vi "COD主界面（列队使用）.vi"() -> (8 "多列列表框":i32(listbox))   [LabVIEW 2016, in "斯坦道CODMn.lvlib"]
uses:
  <vilib>/Plasmionique/MB Master/MB_Master_Serial/MB_Master_Serial.lvclass
  C:/Program Files (x86)/National Instruments/LabVIEW 2016/vi.lib/Plasmionique/MB Master/MB_Master/MB_Master.lvclass
  <vilib>/Analysis/6fits.llb/Curve Fitting Criteria.ctl
  <vilib>/Utility/miscctls.llb/LVPointTypeDef.ctl
  <vilib>/Utility/config.llb/Write Key (Double).vi
  <vilib>/Utility/config.llb/Read Key (Boolean).vi
  <vilib>/Utility/config.llb/Read Key (I32).vi
  <vilib>/Utility/config.llb/Read Key (Double).vi
  <vilib>/Utility/config.llb/Write Key (Boolean).vi
  <vilib>/Utility/config.llb/Write Key (I32).vi
  <vilib>/Waveform/WDTFileIO.llb/Read Waveform from File.vi
  <vilib>/Plasmionique/MB Master/MB Master.lvlib
  <vilib>/ptbypt/NI_PtbyPt.lvlib
  PLC/PLC.lvlib
  <vilib>/Utility/config.llb/NI_LVConfig.lvlib
  <vilib>/Analysis/NI_AALPro.lvlib
panel:
  in  "启用5":bool
  in  "校准5":bool
  in  "泵滴定数5":dbl
  in  "浓度5":dbl
  in  "启用4":bool
  in  "校准4":bool
  in  "泵滴定数4":dbl
  in  "浓度4":dbl
  out "波形时间":timestamp
  in  "历史波形":bool
  out "时间-ORP值":u16[](array[numeric]) caption="数组"
  out "ORP滴定曲线1":u16[](graph)
  out "滴定数-ORP值":u16[](array[numeric]) caption="数组"
  in  "关闭 3":bool
  in  "滴定曲线":bool
  out "ORP滴定曲线2":u16[](graph)
  in  "跨度液浓度":dbl
  out "空白测试标记":bool
  out "跨度核查标记":bool
  out "启动选择 2":u16(ring) items=["水样测试", "标样核查", "零点核查", "跨度核查", "空白测试", "加标回收", "平行样", "校零", "校标"]
  in  "量程选择":enum16{"低量程", "高量程"}(ring)
  out "MB_Serial session":refnum<class "MB_Master_Serial.lvclass">
  in  "手动控制":bool
  in  "选用水样":enum16{"葡萄糖", "草酸钠"}(ring)
  in  "方程系数":cluster{"X^2":dbl, "X":dbl, "b":dbl} {"X^2" format="%#.4g"; "b" format="%#.4g"; "X" format="%#.4g"}
  out "多项式系数1":dbl[](array[numeric]) caption="多项式系数"
  out "XY图":cluster{"X Values":dbl[], "Y Values":dbl[]}[](graph)
  in  "模型":enum32{"线性", "多项式"}(ring)
  out "启动时间":timestamp format="%<%Y/%m/%d %H:%M:%S>T"
  in  "自动切换量程":bool=TRUE
  in  "24H周期设置":bool[](xcontrol)
  in  "关闭 2":bool
  in  "周期设置":bool
  out "文本.文本":string
  out "r^2":dbl format="%.8g"
  out "拟合公式":string
  out "b":dbl format="%#.4g"
  out "K":dbl format="%#.4f"
  out "当前校准":i32
  in  "启用3":bool
  in  "启用2":bool
  in  "启用1":bool
  in  "校准3":bool
  in  "校准2":bool
  in  "校准1":bool
  in  "泵滴定数3":dbl
  in  "泵滴定数2":dbl
  in  "泵滴定数1":dbl
  in  "浓度3":dbl
  in  "浓度2":dbl
  in  "浓度1":dbl
  in  "写入":bool
  out "测量模式数字":i32
  out "零点核查标记":bool
  out "排液故障":bool
  out "进水样超量程":bool
  out "标样核查标记":bool
  out "平行样测量":bool
  out "加标回收测量":bool
  out "质控样测量":bool
  out "待机":bool
  out "校标错误":bool
  out "校零错误":bool
  out "测量错误":bool
  out "草酸钠报警":bool
  out "高锰酸钾报警":bool
  out "加热故障":bool
  out "温控器故障":bool
  out "ORP故障":bool
  out "排液标记":bool
  out "故障标记":bool
  out "校标标记":bool
  out "校零标记":bool
  out "通讯状态":bool
  out "水样测量":bool
  out "读取KB值":bool
  in  "读取":bool
  in  "返回":bool
  in  "校准配置":bool
  in  "修正系数 2":dbl
  in  "浓度 2":dbl
  in  "温度":dbl
  in  "恒温时间":dbl
  in  "基本量程":enum16{"10mL", "20mL"}(ring)
  in  "水样":dbl
  in  "蒸馏水":dbl
  in  "标液":dbl
  in  "质控样":dbl
  in  "加标回收":dbl
  in  "草酸钠":dbl
  in  "高锰酸钾":dbl
  in  "硫酸":dbl
  in  "零点泵计量数 2":dbl
  in  "标度泵计量数 2":dbl
  out "标度滴定值":dbl
  out "零点滴定值":dbl
  in  "保存":bool
  in  "关闭":bool
  out "测量数据区":T1 {"单位" items=["ug/L", "mg/L", "ppm", "mg/m3", "cm", "ppb", "ug/m3", "%", "nmol/mol", "umol/mol", "MPN/L", "MPN/100ml", "ng/m3", "NTU", "无量纲", "ms/cm", "us/cm", "℃", "mV", "万个/L"]}
  out "仪器时间":timestamp format="%<%Y/%m/%d %H:%M:%S>T"
  out "秒":u16
  out "分":u16
  out "COD浓度（mg/L)":dbl format="%.2g"
  out "进样管":dbl
  out "高锰酸钾":dbl
  out "草酸钠":dbl
  out "硫酸":dbl
  out "ORP显示":dbl
  out "温度":dbl
  out "加热":bool
  out "搅拌":bool
  out "进硫酸":bool
  out "进加标回收样":bool
  out "进质控样":bool
  out "进标液":bool
  out "进蒸馏水":bool
  out "进水样":bool
  out "进草酸钠":bool
  out "进高锰酸钾":bool
  in  "定时启动":bool
  in  "启动":bool
  in  "故障清除":bool
  in  "参数配置":bool
  in  "停止":bool
  in  "单步启动":bool
  out "定时时间":dbl
  out "系统时间":timestamp
  in  "时间校准":bool
  in  "枚举":enum16{"读取数据", "写入数据", "读取写入DATABASE", "读取参数"}(ring)
  in  "data in":T2
  out "报警簇":T3
  out "读取参数":u16[](array[numeric])
  out "DATABASE":u16[](array[numeric])
  out "Registers":u16[](array[numeric])
  in  "Slave ID":u8=1
  in  "Serial Config":T4={"baud rate (bps)"=115200, "stop bits"=10, "parity"=0, "flow control"=0, "timeout"=1000, "retries"=1} {"stop bits" items=["1.0"=10, "1.5"=15, "2.0"=20]; "flow control" items=["None", "XON/XOFF", "RTS/CTS", "XON/XOFF & RTS/CTS", "DTR/DSR", "XON/XOFF & DTR/DSR"]; "parity" items=["None", "Odd", "Even", "Mark", "Space"]}
  out "table 输入":string
  out "columns":string[](array[string])
  out "data":T5
  in  "温度 2":dbl
  in  "浓度":dbl
  in  "修正系数":dbl
  in  "标样浓度 2":dbl
  out "模式（受控）":u16
  in  "VISA resource name":refnum<visa-resource-name>="COM4" caption="VISA资源名称"
  # "测量时间："
  # "水样~加标回收"
  # "mV"
  # "℃"
  # "注：遇到加热故障和排液故障时仪器不能正常启动，\n必须排查故障并点击报警清除按钮方可运行。"
  # "mg/L"
  # "校零校标结果"
  # "基本参数设置"
  # "泵计量参数设置"
  # "校零结果："
  # "校零滴定值："
  # "加热恒温温度（℃）："
  # "水样："
  # "高锰酸钾："
  # "校标结果："
  # "标度滴定值："
  # "零点泵计量值："
  # "恒温时间（分钟）："
  # "蒸馏水："
  # "草酸钠："
  # "标度泵计量值："
  # "标准液浓度（mg/L）："
  # "标液："
  # "标样浓度："
  # "硫酸："
  # "修正系数："
  # "质控样："
  # "跨度液浓度："
  # "基本量程（20mL可选）："
  # "加标回收样："
  # "是否启用"
  # "泵滴定数"
  # "浓度"
  # "辅\n助\n计\n算\n区"
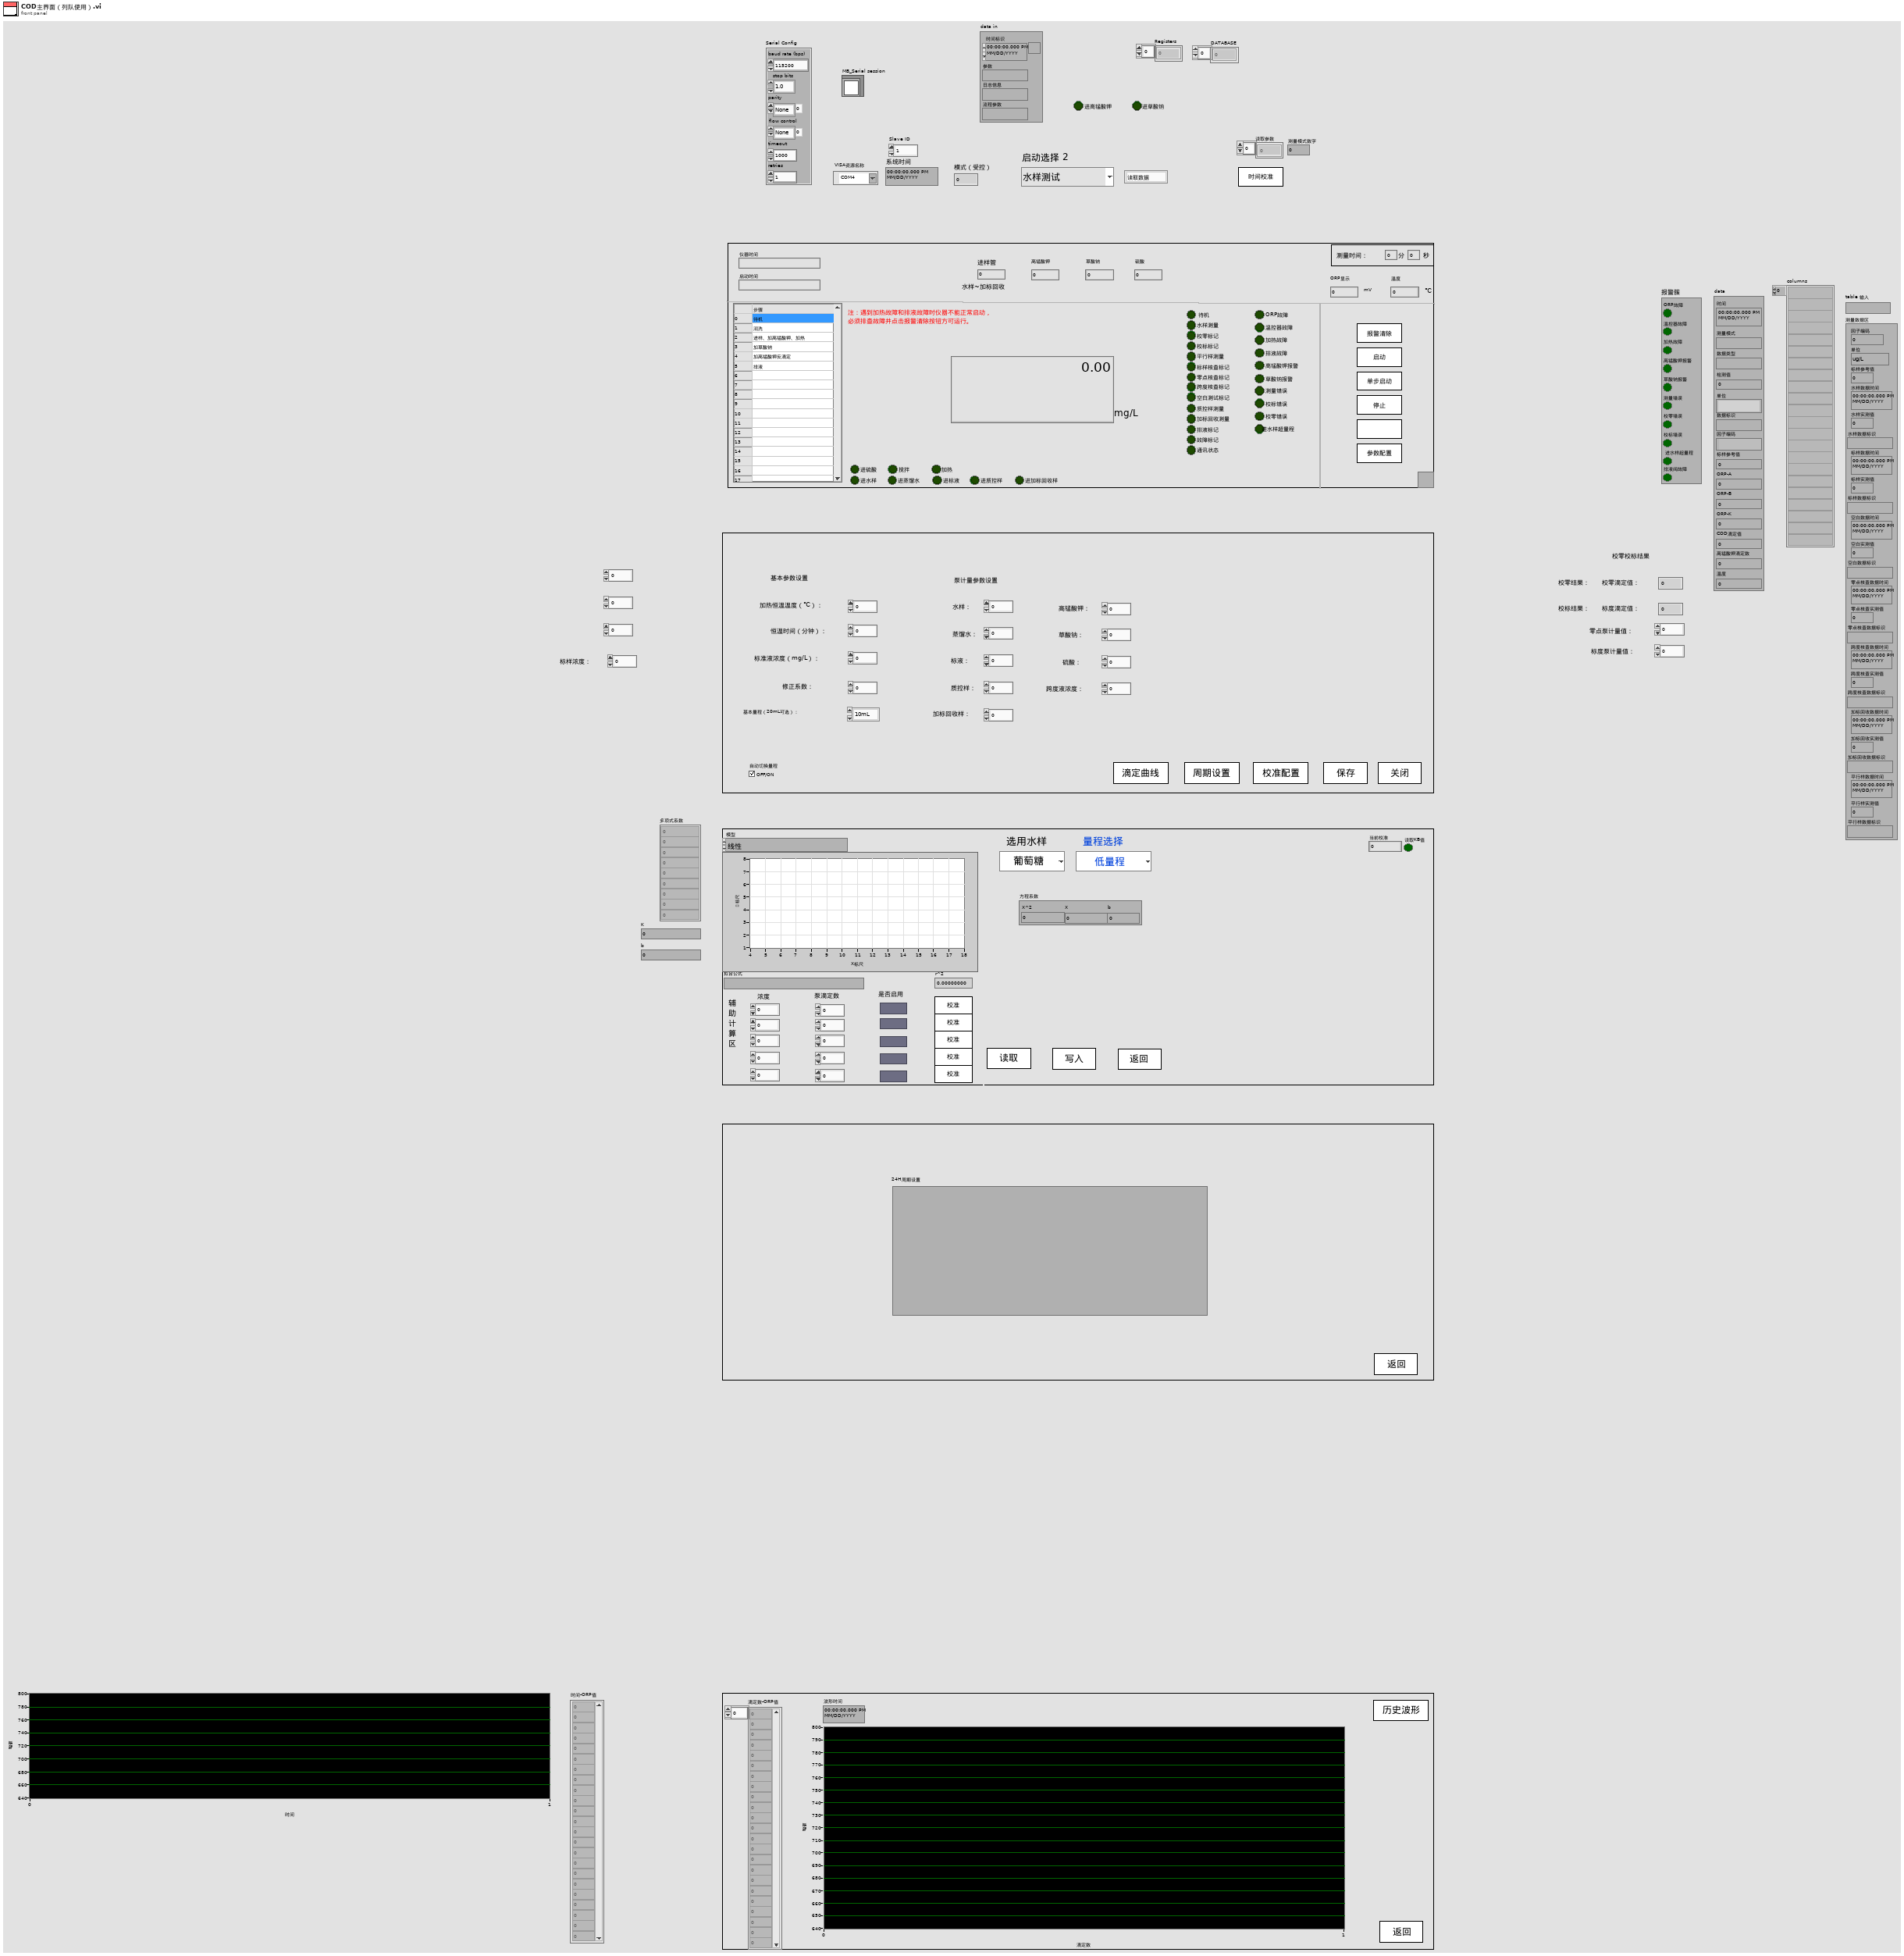
[diagram p1: front panel]
types:
  T1 = cluster{"因子编码":u32, "单位":u16, "标样参考值":sgl, "水样数据时间":timestamp, "水样实测值":sgl, "水样数据标识":string, "标样数据时间":timestamp, "标样实测值":sgl, "标样数据标识":string, "空白数据时间":timestamp, "空白实测值":sgl, "空白数据标识":string, "零点核查数据时间":timestamp, "零点核查实测值":sgl, "零点核查数据标识":string, "跨度核查数据时间":timestamp, "跨度核查实测值":sgl, "跨度核查数据标识":string, "加标回收数据时间":timestamp, "加标回收实测值":sgl, "加标回收数据标识":string, "平行样数据时间":timestamp, "平行样实测值":sgl, "平行样数据标识":string}
  T2 = cluster{"时间标识":timestamp, "参数":string, "日志信息":string, "流程参数":string}
  T3 = cluster{"ORP故障":bool, "温控器故障":bool, "加热故障":bool, "高锰酸钾报警":bool, "草酸钠报警":bool, "测量错误":bool, "校零错误":bool, "校标错误":bool, " 进水样超量程":bool, "排液阀故障":bool}
  T4 = cluster{"baud rate (bps)":u32, "stop bits":u16, "parity":u16, "flow control":u16, "timeout":u32, "retries":i32}
  T5 = cluster{"时间":timestamp, "测量模式":string, "数据类型":string, "检测值":sgl, "单位":string, "数据标识":string, "因子编码":string, "标样参考值":sgl, "ORP-A":sgl, "ORP-B":sgl, "ORP-K":sgl, "COD滴定值":sgl, "高锰酸钾滴定数":sgl, "温度":sgl}
  T6 = cluster{"starting address":u16, "number of holding registers":u16}
  T7 = cluster{"测量模式":enum16{"水样测量", "标样核查", "零点核查", "跨度核查", "空白测试", "加标回收", "平行样", "校零", "校标"}}
  T8 = typedef "LVDateTimeRec.ctl" = cluster{"秒数的小数部分":dbl, "秒":i32, "分":i32, "时":i32, "日":i32, "月":i32, "年":i32, "天数（周）":i32, "天数（年）":i32, "DST":i32}
  T9 = typedef "LVPointTypeDef.ctl" = cluster{"Horizontal":i16, "Vertical":i16}
  T10 = typedef "NI_LVConfig.lvlib/Config Data RefNum.ctl" = refnum<k1>
  T11 = cluster{"时间标识":timestamp, "设备":string, "日志信息":string}
  T12 = typedef "NI_AALPro.lvlib/Curve Fitting Criteria.ctl" = u16
  T13 = cluster{"时间标识":timestamp, "设备":string, "日志信息":string, "流程参数":string}
  T14 = cluster{"数组 2[0]":sgl, "数组 2[1]":sgl, "数组 2[2]":sgl, "数组 2[3]":sgl, "数组 2[4]":sgl, "数组 2[5]":sgl}
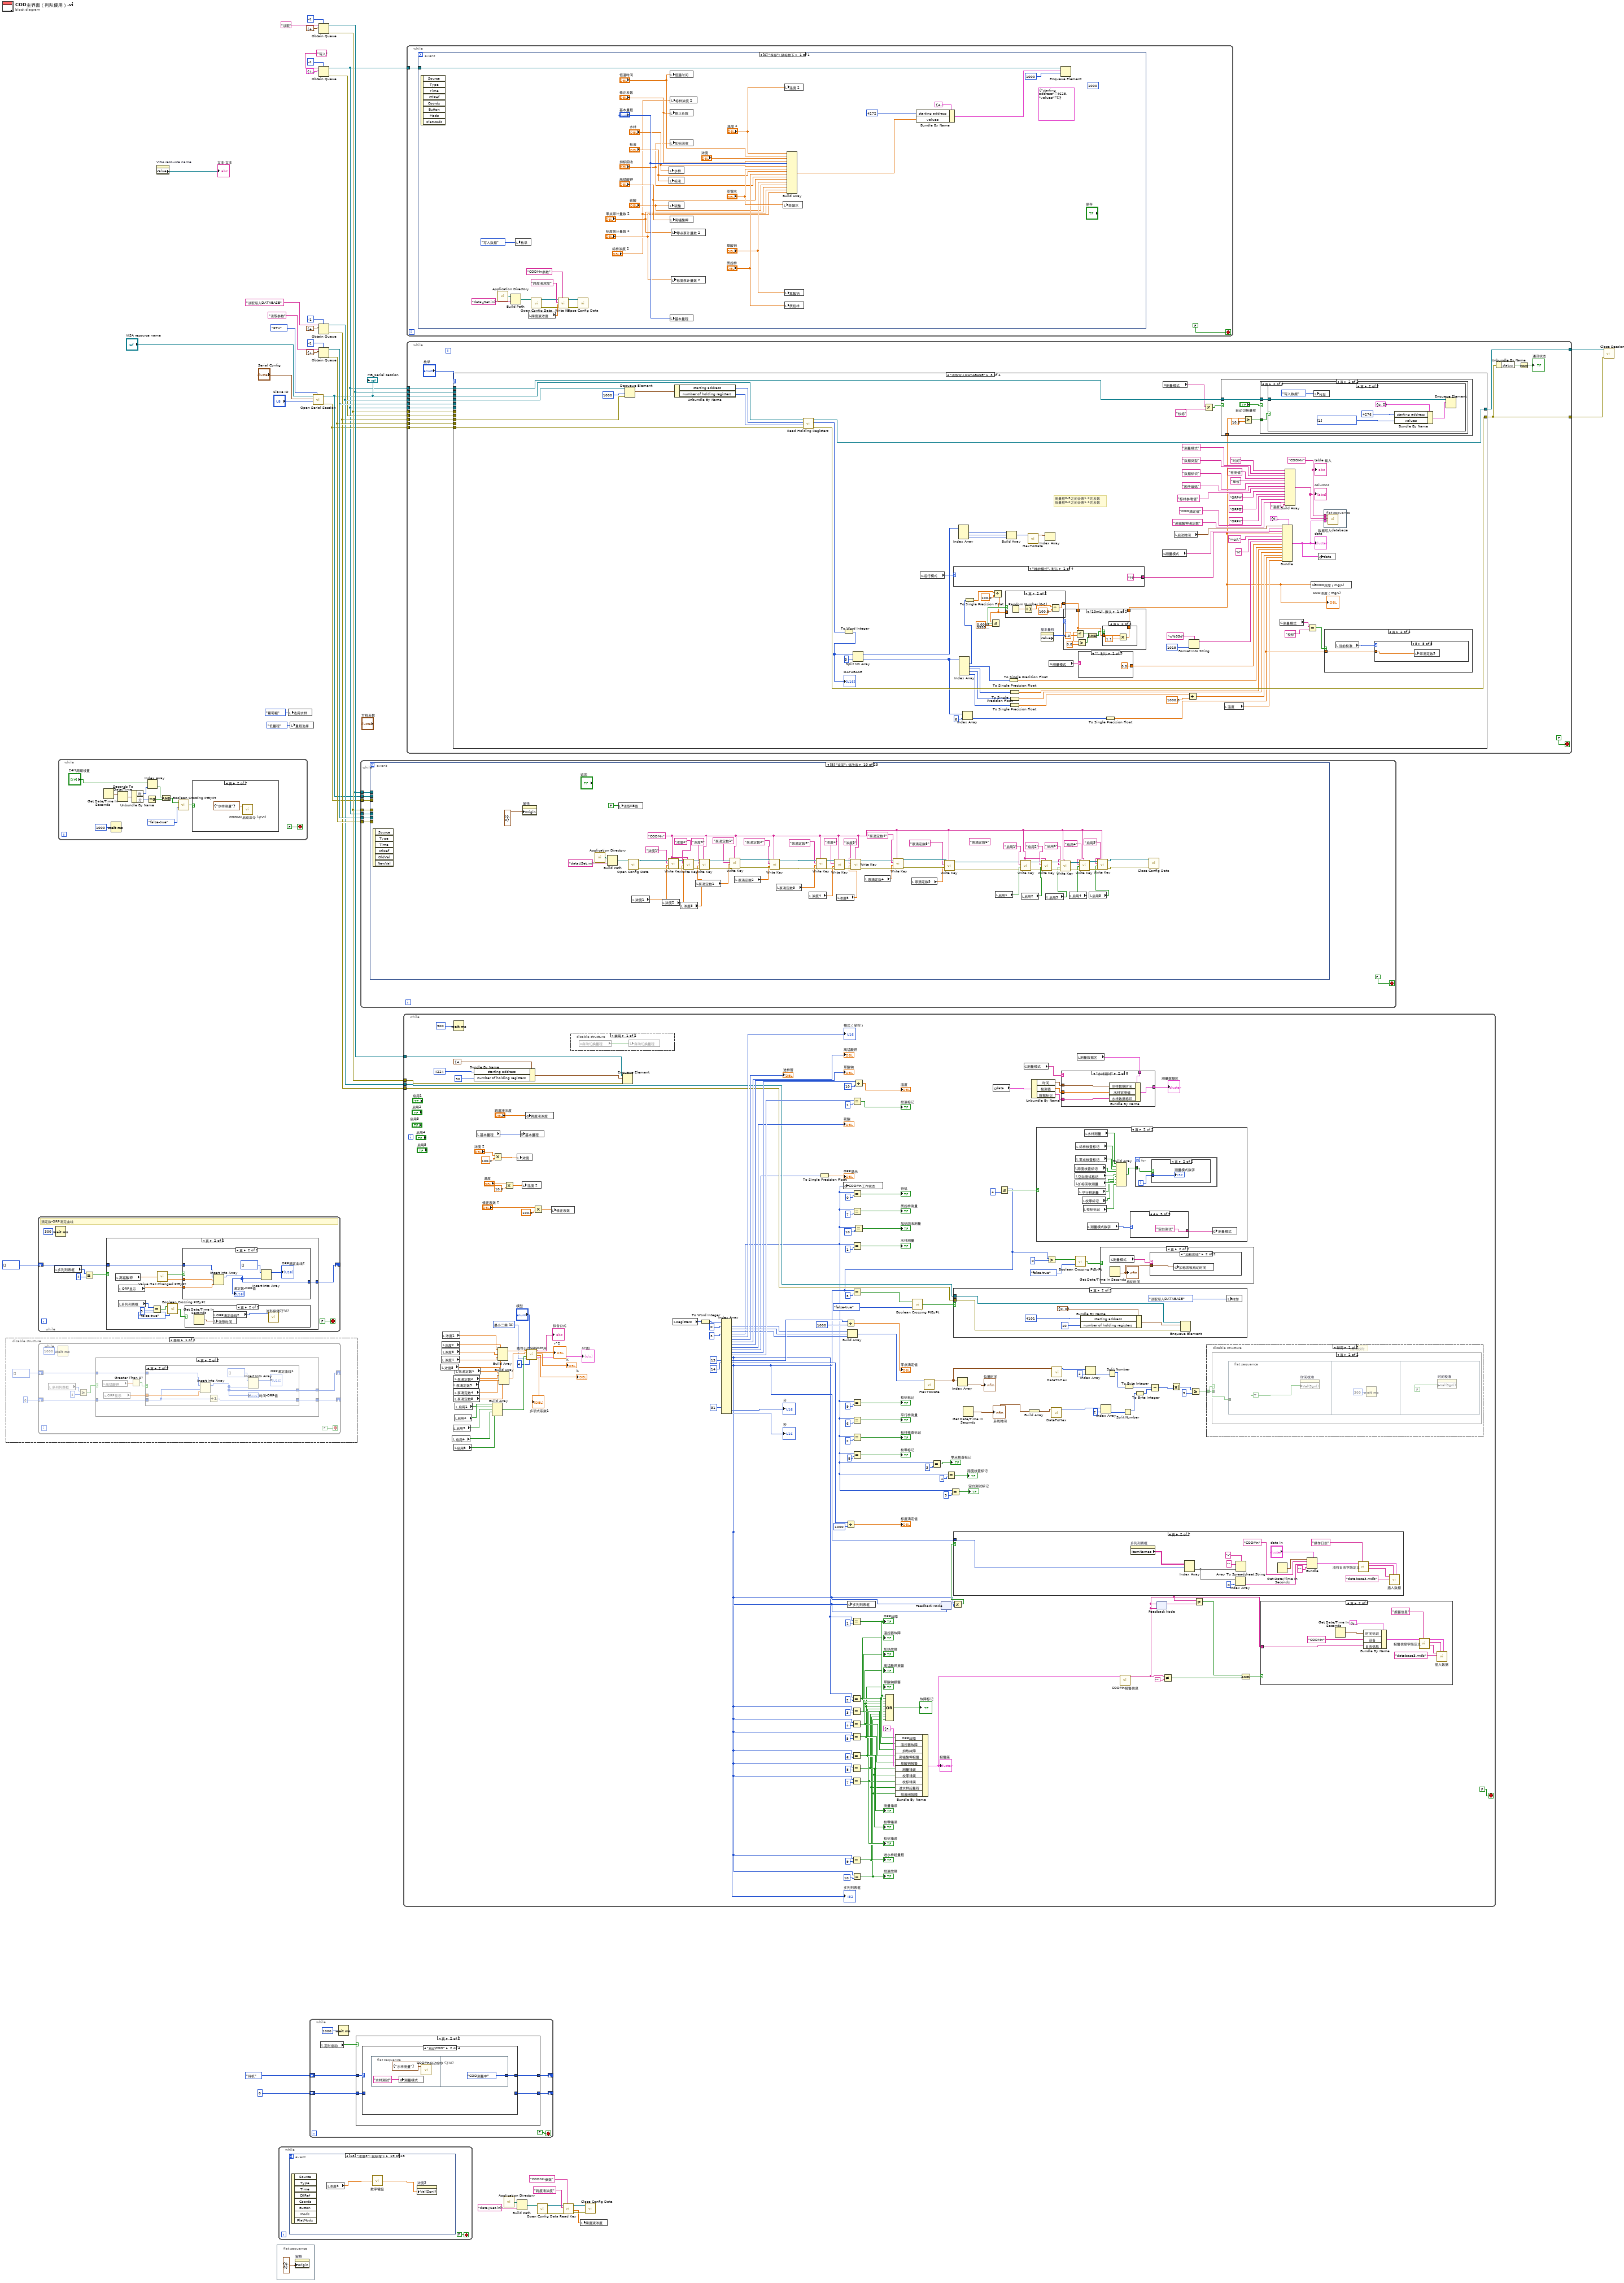
[diagram p0: block diagram]
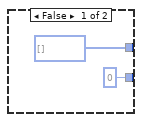
[diagram p2: hidden frame]
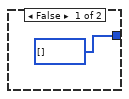
[diagram p5: hidden frame]
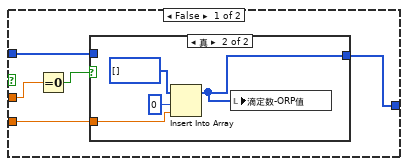
[diagram p7: hidden frame]
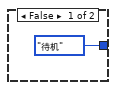
[diagram p10: hidden frame]
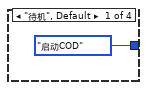
[diagram p11: hidden frame]
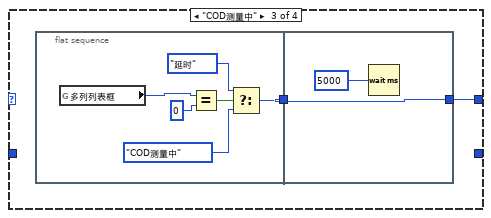
[diagram p12: hidden frame]
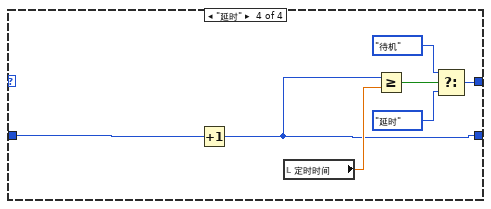
[diagram p13: hidden frame]
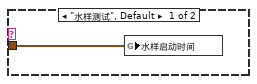
[diagram p18: hidden frame]
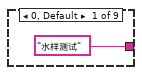
[diagram p20: hidden frame]
diagram:
  n1 = disable-structure shown="禁用" {
    frame Disabled {
      n2 = while {
        shift-right: [w49] -> _
        shift-left: u16[] [] ("ORP滴定曲线") -> [w51]
        shift-right: [w48] -> _
        shift-left: 0 -> [w50]
        stop <- FALSE stop-if-true
        n3 = local read "多列列表框"() -> (w53:i32)
        n4 = Wait (ms)(milliseconds to wait=u32 1000 ("等待时间（毫秒）")) -> ()  [unwired: 1 out]
        n5 = Greater Or Equal?(x=w53, y=4) -> (x >= y?=w52:bool)
        n6 = case shown="真" w52 {
          tunnel: w51 -> [_ w63]
          tunnel: w50 -> [_ w61]
          tunnel: [u16[] [] ("ORP滴定曲线") w59] -> w49
          tunnel: [0 w58] -> w48
          frame False {
          }
          frame True {
            n7 = local read "高锰酸钾"() -> (w62:dbl)
            n8 = local read "ORP显示"() -> (w60:dbl)
            n9 = Greater Than 0?(x=w62) -> (x > 0?=w64:bool)
            n10 = case shown="真" w64 {
              tunnel: w63 -> [w65 w72]
              tunnel: w61 -> [w66 w69]
              tunnel: w60 -> [_ w71]
              tunnel: [w65 w70] -> w59
              tunnel: [w66 w68] -> w58
              frame False {
              }
              frame True {
                n11 = Insert Into Array(array=w72, index=w69, new element=w71) -> (w70:u16[])
                "时间-ORP值" <- w70
                n12 = Increment(x=w69) -> (x+1=w68:i32)
                n13 = Insert Into Array(array=u16[] [] ("ORP滴定曲线"), new element=w70) -> (→"ORP滴定曲线1":u16[])  [unwired: 1 in]
              }
            }
          }
        }
      }
    }
    frame Enabled {
    }
  }
  n14 = while {
    shift-right: [w77] -> _
    shift-left: u16[] [] ("ORP滴定曲线") -> [w78]
    stop <- FALSE stop-if-true
    # "滴定数-ORP滴定曲线"
    n15 = local read "多列列表框"() -> (w76:i32)
    n16 = Wait (ms)(milliseconds to wait=u32 300 ("等待时间（毫秒）")) -> ()  [unwired: 1 out]
    n17 = Greater Or Equal?(x=w76, y=4) -> (x >= y?=w74:bool)
    n18 = case shown="真" w74 {
      tunnel: w78 -> [_ w92]
      tunnel: [u16[] [] ("ORP滴定曲线") w91] -> w77
      frame False {
      }
      frame True {
        n19 = local read "高锰酸钾"() -> (w88:dbl)
        n20 = local read "多列列表框"() -> (w86:i32)
        n21 = local read "ORP显示"() -> (w87:dbl)
        n22 = Equal?(x=w86, y=5) -> (x = y?=w84:bool)
        n23 = call <vilib>:"Value Has Changed PtByPt.vi"("input data point"=w88) -> ("has changed"=w90:bool, "output data point"=w89:dbl)  [unwired: 1 in]
        n24 = call <vilib>:"Boolean Crossing PtByPt.vi"("direction"=enum16{"either", "false-true", "true-false"}."false-true", "input"=w84) -> ("crossing"=w82:bool)  [unwired: 1 in]
        n25 = case shown="真" w90 {
          tunnel: w92 -> [w98 w108]
          tunnel: [w97 w107] -> w91
          tunnel: w89 -> [w99 w106]
          tunnel: w87 -> [w95 w105]
          frame False {
            n26 = Equal To 0?(x=w99) -> (x = 0?=w96:bool)
            n27 = case shown="真" w96 {
              tunnel: [w100 w103] -> w97
              tunnel: w98 -> [w100 _]
              tunnel: w95 -> [_ w102]
              frame False {
              }
              frame True {
                n28 = Insert Into Array(array=u16[] [] ("ORP滴定曲线"), index=0 ("索引"), new element=w102) -> (w103:u16[])
                n29 = local write "滴定数-ORP值"(w103) -> ()
              }
            }
          }
          frame True {
            n30 = Insert Into Array(array=w108, index=w106, new element=w105) -> (w107:u16[])
            "滴定数-ORP值" <- w107
            n31 = Insert Into Array(array=u16[] [] ("ORP滴定曲线"), new element=w107) -> (→"ORP滴定曲线2":u16[])  [unwired: 1 in]
          }
        }
        n32 = case shown="真" w82 {
          frame False {
          }
          frame True {
            n33 = Get Date/Time In Seconds() -> (seconds since 1Jan1904=w93:timestamp)
            n34 = local read "ORP滴定曲线2"() -> (w94:u16[])
            n35 = local write "波形时间"(w93) -> ()
            n36 = call "波形存储(子VI).vi"("ORP滴定曲线"=w94) -> ()  [unwired: 11 in]
          }
        }
      }
    }
  }
  n37 = while {
    stop <- FALSE stop-if-true
    n38 = Get Date/Time In Seconds() -> (seconds since 1Jan1904=w122:timestamp)
    n39 = Wait (ms)(milliseconds to wait=u32 1000 ("等待时间（毫秒）")) -> ()  [unwired: 1 out]
    n40 = Seconds To Date/Time(time stamp (now)=w122) -> (date time rec=w121:T8)  [unwired: 1 in]
    n41 = Unbundle By Name(w121) -> ("时"=w118:i32, "分"=w120:i32)
    n42 = Equal To 0?(x=w120) -> (x = 0?=w119:bool)
    n43 = Index Array(array="24H周期设置", index=w118) -> (element=w117:bool)
    n44 = And(x=w117, y=w119) -> (x .and. y?=w115:bool)
    n45 = call <vilib>:"Boolean Crossing PtByPt.vi"("direction"=enum16{"either", "false-true", "true-false"}."false-true", "input"=w115) -> ("crossing"=w114:bool)  [unwired: 1 in]
    n46 = case shown="真" w114 {
      frame False {
      }
      frame True {
        n47 = call "CODMn启动命令 (子VI).vi"("启动测量模式"=T7 {"测量模式"=enum."水样测量"}) -> ()  [unwired: 11 in]
      }
    }
  }
  n48 = property on="VISA resource name" class="VISAName"() -> ("Value"=→"文本.文本":refnum<visa-resource-name>)  [unwired: 2 in, 2 out]
  n49 = flat-sequence {
    frame #0 {
      n50 = property on="窗格" class="Pane"("Origin"=T9 {"Horizontal"=0, "Vertical"=0} ("原点")) -> ()  [unwired: 2 in, 2 out]
    }
  }
  n51 = while {
    stop <- FALSE stop-if-true
    n52 = event shown="[18] \"浓度3\": 鼠标按下" {
      selector: _ -> [_ _ _ _ _ _ _ _ _ _ _ _ _ _ _ _ _ _ _ _ _ _ _ _ _ _ _ _]
      dyn-events: _ -> [_ _ _ _ _ _ _ _ _ _ _ _ _ _ _ _ _ _ _ _ _ _ _ _ _ _ _ _]
      timeout: _ -> [_ _ _ _ _ _ _ _ _ _ _ _ _ _ _ _ _ _ _ _ _ _ _ _ _ _ _ _]
      event Timeout {
        n53 = event-data() -> ()  [unwired: 1 in, 3 out]
      }
      event "温度": Mouse Down {
        n54 = event-data() -> ()  [unwired: 1 in, 8 out]
        n55 = local read "温度"() -> (w127:dbl)
        n56 = call "数字键盘.vi"("OldNumber"=w127) -> ("NewNumber"=w126:sgl)
        n57 = local write "温度"(w126) -> ()
      }
      event "恒温时间": Mouse Down {
        n58 = event-data() -> ()  [unwired: 1 in, 8 out]
        n59 = local read "恒温时间"() -> (w128:dbl)
        n60 = call "数字键盘.vi"("OldNumber"=w128) -> ("NewNumber"=w129:sgl)
        n61 = local write "恒温时间"(w129) -> ()
      }
      event "浓度 2": Mouse Down {
        n62 = event-data() -> ()  [unwired: 1 in, 8 out]
        n63 = local read "浓度 2"() -> (w131:dbl)
        n64 = call "数字键盘.vi"("OldNumber"=w131) -> ("NewNumber"=w130:sgl)
        n65 = local write "浓度 2"(w130) -> ()
      }
      event "修正系数 2": Mouse Down {
        n66 = event-data() -> ()  [unwired: 1 in, 8 out]
        n67 = local read "修正系数 2"() -> (w132:dbl)
        n68 = call "数字键盘.vi"("OldNumber"=w132) -> ("NewNumber"=w133:sgl)
        n69 = local write "修正系数 2"(w133) -> ()
      }
      event "水样": Mouse Down {
        n70 = event-data() -> ()  [unwired: 1 in, 8 out]
        n71 = local read "水样"() -> (w134:dbl)
        n72 = call "数字键盘.vi"("OldNumber"=w134) -> ("NewNumber"=w135:sgl)
        n73 = local write "水样"(w135) -> ()
      }
      event "蒸馏水": Mouse Down {
        n74 = event-data() -> ()  [unwired: 1 in, 8 out]
        n75 = local read "蒸馏水"() -> (w136:dbl)
        n76 = call "数字键盘.vi"("OldNumber"=w136) -> ("NewNumber"=w137:sgl)
        n77 = local write "蒸馏水"(w137) -> ()
      }
      event "标液": Mouse Down {
        n78 = event-data() -> ()  [unwired: 1 in, 8 out]
        n79 = local read "标液"() -> (w138:dbl)
        n80 = call "数字键盘.vi"("OldNumber"=w138) -> ("NewNumber"=w139:sgl)
        n81 = local write "标液"(w139) -> ()
      }
      event "质控样": Mouse Down {
        n82 = event-data() -> ()  [unwired: 1 in, 8 out]
        n83 = local read "质控样"() -> (w140:dbl)
        n84 = call "数字键盘.vi"("OldNumber"=w140) -> ("NewNumber"=w141:sgl)
        n85 = local write "质控样"(w141) -> ()
      }
      event "加标回收": Mouse Down {
        n86 = event-data() -> ()  [unwired: 1 in, 8 out]
        n87 = local read "加标回收"() -> (w142:dbl)
        n88 = call "数字键盘.vi"("OldNumber"=w142) -> ("NewNumber"=w143:sgl)
        n89 = local write "加标回收"(w143) -> ()
      }
      event "草酸钠": Mouse Down {
        n90 = event-data() -> ()  [unwired: 1 in, 8 out]
        n91 = local read "草酸钠"() -> (w144:dbl)
        n92 = call "数字键盘.vi"("OldNumber"=w144) -> ("NewNumber"=w145:sgl)
        n93 = local write "草酸钠"(w145) -> ()
      }
      event "高锰酸钾": Mouse Down {
        n94 = event-data() -> ()  [unwired: 1 in, 8 out]
        n95 = local read "高锰酸钾"() -> (w146:dbl)
        n96 = call "数字键盘.vi"("OldNumber"=w146) -> ("NewNumber"=w147:sgl)
        n97 = local write "高锰酸钾"(w147) -> ()
      }
      event "硫酸": Mouse Down {
        n98 = event-data() -> ()  [unwired: 1 in, 8 out]
        n99 = local read "硫酸"() -> (w148:dbl)
        n100 = call "数字键盘.vi"("OldNumber"=w148) -> ("NewNumber"=w149:sgl)
        n101 = local write "硫酸"(w149) -> ()
      }
      event "零点泵计量数 2": Mouse Down {
        n102 = event-data() -> ()  [unwired: 1 in, 8 out]
        n103 = local read "零点泵计量数 2"() -> (w150:dbl)
        n104 = call "数字键盘.vi"("OldNumber"=w150) -> ("NewNumber"=w151:sgl)
        n105 = local write "零点泵计量数 2"(w151) -> ()
      }
      event "标度泵计量数 2": Mouse Down {
        n106 = event-data() -> ()  [unwired: 1 in, 8 out]
        n107 = local read "标度泵计量数 2"() -> (w152:dbl)
        n108 = call "数字键盘.vi"("OldNumber"=w152) -> ("NewNumber"=w153:sgl)
        n109 = local write "标度泵计量数 2"(w153) -> ()
      }
      event "标样浓度 2": Mouse Down {
        n110 = event-data() -> ()  [unwired: 1 in, 8 out]
        n111 = local read "标样浓度 2"() -> (w154:dbl)
        n112 = call "数字键盘.vi"("OldNumber"=w154) -> ("NewNumber"=w155:sgl)
        n113 = local write "标样浓度 2"(w155) -> ()
      }
      event "浓度1": Mouse Down {
        n114 = event-data() -> ()  [unwired: 1 in, 8 out]
        n115 = local read "浓度1"() -> (w157:dbl)
        n116 = call "数字键盘.vi"("OldNumber"=w157) -> ("NewNumber"=w156:sgl)
        n117 = property on="浓度1" class="DigNum (严格)"("Val(Sgnl)"=w156) -> ()  [unwired: 2 in, 2 out]
      }
      event "浓度2": Mouse Down {
        n118 = event-data() -> ()  [unwired: 1 in, 8 out]
        n119 = local read "浓度2"() -> (w159:dbl)
        n120 = call "数字键盘.vi"("OldNumber"=w159) -> ("NewNumber"=w158:sgl)
        n121 = property on="浓度2" class="DigNum (严格)"("Val(Sgnl)"=w158) -> ()  [unwired: 2 in, 2 out]
      }
      event "浓度3": Mouse Down {
        n122 = event-data() -> ()  [unwired: 1 in, 8 out]
        n123 = local read "浓度3"() -> (w161:dbl)
        n124 = call "数字键盘.vi"("OldNumber"=w161) -> ("NewNumber"=w160:sgl)
        n125 = property on="浓度3" class="DigNum (严格)"("Val(Sgnl)"=w160) -> ()  [unwired: 2 in, 2 out]
      }
      event "浓度4": Mouse Down {
        n126 = event-data() -> ()  [unwired: 1 in, 8 out]
        n127 = local read "浓度4"() -> (w163:dbl)
        n128 = call "数字键盘.vi"("OldNumber"=w163) -> ("NewNumber"=w162:sgl)
        n129 = property on="浓度4" class="DigNum (严格)"("Val(Sgnl)"=w162) -> ()  [unwired: 2 in, 2 out]
      }
      event "浓度5": Mouse Down {
        n130 = event-data() -> ()  [unwired: 1 in, 8 out]
        n131 = local read "浓度5"() -> (w165:dbl)
        n132 = call "数字键盘.vi"("OldNumber"=w165) -> ("NewNumber"=w164:sgl)
        n133 = property on="浓度5" class="DigNum (严格)"("Val(Sgnl)"=w164) -> ()  [unwired: 2 in, 2 out]
      }
      event "跨度液浓度": Mouse Down {
        n134 = event-data() -> ()  [unwired: 1 in, 8 out]
        n135 = local read "跨度液浓度"() -> (w167:dbl)
        n136 = call "数字键盘.vi"("OldNumber"=w167) -> ("NewNumber"=w166:sgl)
        n137 = property on="跨度液浓度" class="DigNum (严格)"("Val(Sgnl)"=w166) -> ()  [unwired: 2 in, 2 out]
      }
      event "跨度液浓度": Value Change {
        n138 = event-data() -> ()  [unwired: 1 in, 6 out]
        n139 = call <vilib>:"Application Directory.vi"() -> ("Application Directory"=w171:path)
        n140 = Build Path(base path=w171, name or relative path="data\\Set.ini" ("名称或相对路径")) -> (appended path=w173:path)
        n141 = local read "跨度液浓度"() -> (w168:dbl)
        n142 = call <vilib>:"Open Config Data.vi"("configuration file path"=w173) -> ("error out"=w175:errorcluster, "refnum"=w174:T10)  [unwired: 8 in, 1 out]
        n143 = call-poly <vilib>:"Write Key.vi"("section"="CODMn参数" ("key"), "error in (no error)"=w175, "value"=w168, "key"="跨度液浓度", "refnum"=w174) -> ("error out"=w177:errorcluster, "refnum out"=w176:T10)  [unwired: 4 in, 1 out]
        n144 = call <vilib>:"Close Config Data.vi"("error in (no error)"=w177, "refnum"=w176) -> ()  [unwired: 8 in, 2 out]
      }
      event "泵滴定数1": Mouse Down {
        n145 = event-data() -> ()  [unwired: 1 in, 8 out]
        n146 = local read "泵滴定数1"() -> (w179:dbl)
        n147 = call "数字键盘.vi"("OldNumber"=w179) -> ("NewNumber"=w178:sgl)
        n148 = property on="泵滴定数1" class="DigNum (严格)"("Val(Sgnl)"=w178) -> ()  [unwired: 2 in, 2 out]
      }
      event "泵滴定数2": Mouse Down {
        n149 = event-data() -> ()  [unwired: 1 in, 8 out]
        n150 = local read "泵滴定数2"() -> (w181:dbl)
        n151 = call "数字键盘.vi"("OldNumber"=w181) -> ("NewNumber"=w180:sgl)
        n152 = property on="泵滴定数2" class="DigNum (严格)"("Val(Sgnl)"=w180) -> ()  [unwired: 2 in, 2 out]
      }
      event "泵滴定数3": Mouse Down {
        n153 = event-data() -> ()  [unwired: 1 in, 8 out]
        n154 = local read "泵滴定数3"() -> (w183:dbl)
        n155 = call "数字键盘.vi"("OldNumber"=w183) -> ("NewNumber"=w182:sgl)
        n156 = property on="泵滴定数3" class="DigNum (严格)"("Val(Sgnl)"=w182) -> ()  [unwired: 2 in, 2 out]
      }
      event "泵滴定数4": Mouse Down {
        n157 = event-data() -> ()  [unwired: 1 in, 8 out]
        n158 = local read "泵滴定数4"() -> (w185:dbl)
        n159 = call "数字键盘.vi"("OldNumber"=w185) -> ("NewNumber"=w184:sgl)
        n160 = property on="泵滴定数4" class="DigNum (严格)"("Val(Sgnl)"=w184) -> ()  [unwired: 2 in, 2 out]
      }
      event "泵滴定数5": Mouse Down {
        n161 = event-data() -> ()  [unwired: 1 in, 8 out]
        n162 = local read "泵滴定数5"() -> (w187:dbl)
        n163 = call "数字键盘.vi"("OldNumber"=w187) -> ("NewNumber"=w186:sgl)
        n164 = property on="泵滴定数5" class="DigNum (严格)"("Val(Sgnl)"=w186) -> ()  [unwired: 2 in, 2 out]
      }
    }
  }
  n165 = local write "选用水样"(enum16{"葡萄糖", "草酸钠"}."葡萄糖" ("选用水样")) -> ()
  n166 = local write "量程选择"(enum16{"低量程", "高量程"}."低量程" ("量程选择")) -> ()
  n167 = while {
    shift-right: [w189] -> _
    shift-left: enum16{"待机", "启动COD", "COD测量中", "延时"}."待机" -> [w191]
    shift-right: [w188] -> _
    shift-left: 0 -> [w190]
    stop <- FALSE stop-if-true
    n168 = local read "定时启动"() -> (w193:bool)
    n169 = Wait (ms)(milliseconds to wait=u32 1000 ("等待时间（毫秒）")) -> ()  [unwired: 1 out]
    n170 = case shown="真" w193 {
      tunnel: w191 -> [_ w199]
      tunnel: w190 -> [_ w198]
      tunnel: [enum16{"待机", "启动COD", "COD测量中", "延时"}."待机" w197] -> w189
      tunnel: [_ w196] -> w188
      frame False {
      }
      frame True {
        n171 = case shown="\"启动COD\"" w199 {
          tunnel: w198 -> [_ _ _ w221]
          tunnel: [enum16{"待机", "启动COD", "COD测量中", "延时"}."启动COD" w201 w206 w215] -> w197
          tunnel: [_ _ _ w218] -> w196
          frame "待机", Default {
          }
          frame "启动COD" {
            n172 = flat-sequence {
              tunnel: [enum16{"待机", "启动COD", "COD测量中", "延时"}."COD测量中"] -> w201
              frame #0 {
                n173 = global write "COD测量模式全局.vi" "测量模式"("水样测试" ("测量模式")) -> ()
                n174 = call "CODMn启动命令 (子VI).vi"("启动测量模式"=T7 {"测量模式"=enum."水样测量"}) -> ()  [unwired: 11 in]
              }
              frame #1 {
              }
            }
          }
          frame "COD测量中" {
            n175 = flat-sequence {
              tunnel: [w207] -> w205
              tunnel: [w214] -> w206
              tunnel: w205 -> [w214]
              frame #0 {
                n176 = global read "运行时序全局变量.vi" "多列列表框"() -> (w212:i32)
                n177 = Equal?(x=w212, y=0) -> (x = y?=w210:bool)
                n178 = Select(t=enum16{"待机", "启动COD", "COD测量中", "延时"}."延时", s=w210, f=enum16{"待机", "启动COD", "COD测量中", "延时"}."COD测量中") -> (s? t:f=w207:enum16{"待机", "启动COD", "COD测量中", "延时"})
              }
              frame #1 {
                n179 = Wait (ms)(milliseconds to wait=u32 5000 ("等待时间（毫秒）")) -> ()  [unwired: 1 out]
              }
            }
          }
          frame "延时" {
            n180 = Increment(x=w221) -> (x+1=w218:i32)
            n181 = local read "定时时间"() -> (w220:dbl)
            n182 = Greater Or Equal?(x=w218, y=w220) -> (x >= y?=w219:bool)
            n183 = Select(t=enum16{"待机", "启动COD", "COD测量中", "延时"}."待机", s=w219, f=enum16{"待机", "启动COD", "COD测量中", "延时"}."延时") -> (s? t:f=w215:enum16{"待机", "启动COD", "COD测量中", "延时"})
          }
        }
      }
    }
  }
  n184 = call <vilib>:"Open Serial Session.vi"("Mode (RTU)"=enum16{"RTU", "ASCII"}."RTU", "Slave ID"="Slave ID", "Serial Config"="Serial Config", "VISA Resource"="VISA resource name") -> ("Error out"=w18:errorcluster, "MB_Serial session"=w19:refnum<class "MB_Master_Serial.lvclass">)  [unwired: 6 in]
  "MB_Serial session" <- w19
  n185 = Obtain Queue(max queue size (-1, unlimited)=-1 ("队列最大值（-1，无限）"), name (unnamed)="读取" ("名称（未命名）"), element data type=T6 {"starting address"=4224, "number of holding registers"=16}) -> (queue out=w34:refnum<queue>, error out=w33:errorcluster)  [unwired: 2 in, 1 out]
  n186 = Obtain Queue(max queue size (-1, unlimited)=-1 ("队列最大值（-1，无限）"), name (unnamed)="写入" ("名称（未命名）"), element data type=cluster{"starting address":u16, "values":u16[]} {"starting address"=4272, "values"=[]}) -> (queue out=w15:refnum<queue>, error out=w20:errorcluster)  [unwired: 2 in, 1 out]
  n187 = Obtain Queue(max queue size (-1, unlimited)=-1 ("队列最大值（-1，无限）"), name (unnamed)="读取写入DATABASE" ("名称（未命名）"), element data type=T6 {"starting address"=4224, "number of holding registers"=16}) -> (queue out=w22:refnum<queue>, error out=w21:errorcluster)  [unwired: 2 in, 1 out]
  n188 = Obtain Queue(max queue size (-1, unlimited)=-1 ("队列最大值（-1，无限）"), name (unnamed)="读取参数" ("名称（未命名）"), element data type=T6 {"starting address"=4224, "number of holding registers"=16}) -> (queue out=w27:refnum<queue>, error out=w26:errorcluster)  [unwired: 2 in, 1 out]
  n189 = while {
    tunnel: w34 -> [w229]
    tunnel: w33 -> [w228]
    tunnel: w15 -> [w227]
    tunnel: w27 -> [w226]
    tunnel: w26 -> [w225]
    tunnel: w19 -> [w223]
    tunnel: w18 -> [w222]
    stop <- FALSE stop-if-true
    n190 = event shown="[9] \"返回\": 值改变" {
      selector: _ -> [_ _ _ _ _ _ _ _ _ _ _ _ _ _ _ _ _ _ _ _ _ _ _]
      dyn-events: _ -> [_ _ _ _ _ _ _ _ _ _ _ _ _ _ _ _ _ _ _ _ _ _ _]
      timeout: _ -> [_ _ _ _ _ _ _ _ _ _ _ _ _ _ _ _ _ _ _ _ _ _ _]
      tunnel: w229 -> [_ _ _ _ _ _ _ _ _ _ _ _ _ _ _ _ _ _ _ _ _ _ _]
      tunnel: w228 -> [_ _ _ _ _ _ _ _ _ _ _ _ _ _ _ _ _ _ _ _ _ _ _]
      tunnel: w227 -> [w237 w270 w307 _ _ _ _ _ _ _ _ _ w660 w674 _ w682 _ _ _ _ w860 _ _]
      tunnel: w226 -> [_ _ _ _ w326 _ _ _ _ _ _ _ _ _ _ _ _ _ _ w852 _ _ _]
      tunnel: w225 -> [_ _ _ _ w325 _ _ _ _ _ _ _ _ _ _ _ _ _ _ w851 _ _ _]
      tunnel: w223 -> [_ _ _ w313 _ _ _ _ _ _ _ w659 _ _ _ _ _ _ _ _ _ _ _]
      tunnel: w222 -> [_ _ _ w312 _ _ _ _ _ _ _ w658 _ _ _ _ _ _ _ _ _ _ _]
      event "单步启动": Mouse Down {
        n191 = event-data() -> ()  [unwired: 1 in, 8 out]
        n192 = call "单步启动选择对话框.vi"() -> ("启动选择2"=w230:u16)  [unwired: 10 in, 1 out]
        n193 = case shown="12, 默认" w230 {
          tunnel: [u16 4610 ("address") u16 4610 ("address") u16 4610 ("address") u16 4610 ("address") u16 4610 ("address") u16 4610 ("address") u16 4610 ("address") u16 4610 ("address") u16 4610 ("address") u16 4610 ("address") u16 4610 ("address") u16 4610 ("address") u16 4610 ("address")] -> w236
          tunnel: [u16 1 ("address") u16 2 ("address") u16 3 ("address") u16 4 ("address") u16 5 ("address") u16 6 ("address") u16 7 ("address") u16 8 ("address") u16 9 ("holding register value") u16 10 ("holding register value") u16 11 ("holding register value") u16 12 ("address") u16 0 ("address")] -> w233
          frame 0 {
          }
          frame 1 {
          }
          frame 2 {
          }
          frame 3 {
          }
          frame 4 {
          }
          frame 5 {
          }
          frame 6 {
          }
          frame 7 {
          }
          frame 8 {
          }
          frame 9 {
          }
          frame 10 {
          }
          frame 11 {
          }
          frame 12, Default {
          }
        }
        n194 = local write "枚举"(enum16{"读取数据", "写入数据", "读取写入DATABASE", "读取参数"}."写入数据" ("枚举")) -> ()
        n195 = Insert Into Array(array=u16[] [] ("values"), index=0 ("索引"), new element=w233) -> (w232:u16[])
        n196 = Bundle By Name(cluster=cluster{"starting address":u16, "values":u16[]} {"starting address"=0, "values"=[]}, "starting address"=w236, "values"=w232) -> (w238:cluster{"starting address":u16, "values":u16[]})
        n197 = Enqueue Element(queue=w237, element=w238) -> ()  [unwired: 2 in, 3 out]
      }
      event "启动": Mouse Down {
        n198 = event-data() -> ()  [unwired: 1 in, 8 out]
        n199 = flat-sequence {
          tunnel: w270 -> [w273]
          tunnel: [w273] -> w269
          tunnel: [w272] -> w266
          tunnel: w269 -> [w276]
          tunnel: [w276] -> w268
          tunnel: [w274] -> w267
          tunnel: w266 -> [w274]
          tunnel: w268 -> [w278]
          tunnel: w267 -> [w277]
          frame #0 {
            n200 = call "启动测量模式选择对话框.vi"() -> ("启动选择 2"=w272:u16)  [unwired: 11 in]
            "启动选择 2" <- w272
          }
          frame #1 {
            n201 = property on="启动选择 2" class="Ring (严格)"() -> ("RingText.Text"=w275:string)  [unwired: 2 in, 2 out]
            n202 = global write "COD测量模式全局.vi" "测量模式"(w275) -> ()
          }
          frame #2 {
            n203 = case shown="9, 默认" w277 {
              tunnel: [u16 4608 ("address") u16 4608 ("address") u16 4608 ("address") u16 4608 ("address") u16 4608 ("address") u16 4608 ("address") u16 4608 ("address") u16 4608 ("address") u16 4608 ("address") u16 4608 ("address")] -> w279
              tunnel: [u16 1 ("address") u16 2 ("address") u16 3 ("address") u16 4 ("address") u16 5 ("address") u16 7 ("address") u16 6 ("address") u16 8 ("address") u16 9 ("address") u16 0 ("address")] -> w280
              frame 0 {
              }
              frame 1 {
              }
              frame 2 {
              }
              frame 3 {
              }
              frame 4 {
              }
              frame 5 {
              }
              frame 6 {
              }
              frame 7 {
              }
              frame 8 {
              }
              frame 9, Default {
              }
            }
            n204 = Insert Into Array(array=u16[] [] ("values"), index=0 ("索引"), new element=w280) -> (w285:u16[])
            n205 = Bundle By Name(cluster=cluster{"starting address":u16, "values":u16[]} {"starting address"=0, "values"=[]}, "starting address"=w279, "values"=w285) -> (w282:cluster{"starting address":u16, "values":u16[]})
            n206 = Enqueue Element(queue=w278, element=w282) -> ()  [unwired: 2 in, 3 out]
          }
        }
        n207 = local write "枚举"(enum16{"读取数据", "写入数据", "读取写入DATABASE", "读取参数"}."写入数据" ("枚举")) -> ()
      }
      event "停止": Value Change {
        n208 = event-data() -> ()  [unwired: 1 in, 6 out]
        n209 = local write "枚举"(enum16{"读取数据", "写入数据", "读取写入DATABASE", "读取参数"}."写入数据" ("枚举")) -> ()
        n210 = Bundle By Name(cluster=cluster{"starting address":u16, "values":u16[]} {"starting address"=0, "values"=[]}, "starting address"=u16 4608, "values"=u16[] [11]) -> (w309:cluster{"starting address":u16, "values":u16[]})
        n211 = Enqueue Element(queue=w307, element=w309) -> ()  [unwired: 2 in, 3 out]
      }
      event "手动控制": Value Change {
        n212 = event-data() -> ()  [unwired: 1 in, 6 out]
        n213 = call "CODMn手动控制框.vi"("Error in"=w312, "MB_Serial session"=w313) -> ()  [unwired: 10 in]
      }
      event "参数配置": Value Change {
        n214 = event-data() -> ()  [unwired: 1 in, 6 out]
        n215 = property on="窗格" class="Pane"("Origin"=T9 {"Horizontal"=0, "Vertical"=650} ("原点")) -> ()  [unwired: 2 in, 2 out]
        n216 = Bundle By Name(cluster=T6 {"starting address"=0, "number of holding registers"=0}, "starting address"=u16 4240, "number of holding registers"=u16 16) -> (w333:T6)
        n217 = local write "读取KB值"(FALSE ("读取KB值")) -> ()
        n218 = local write "枚举"(enum16{"读取数据", "写入数据", "读取写入DATABASE", "读取参数"}."读取参数" ("枚举")) -> ()
        n219 = Flush Queue(queue=w326, error in (no error)=w325) -> (queue out=w329:refnum<queue>, error out=w328:errorcluster)  [unwired: 1 out]
        n220 = Enqueue Element(queue=w329, element=w333, error in (no error)=w328) -> ()  [unwired: 1 in, 3 out]
        n221 = call <vilib>:"Application Directory.vi"() -> ("Application Directory"=w321:path)
        n222 = Build Path(base path=w321, name or relative path="data\\Set.ini" ("名称或相对路径")) -> (appended path=w319:path)
        n223 = call <vilib>:"Open Config Data.vi"("configuration file path"=w319) -> ("error out"=w322:errorcluster, "refnum"=w323:T10)  [unwired: 8 in, 1 out]
        n224 = call-poly <vilib>:"Read Key.vi"("section"="CODMn是否切换量程" ("key"), "error in (no error)"=w322, "key"="自动切换量程", "refnum"=w323) -> ("error out"=w315:errorcluster, "value"=w314:bool, "refnum out"=w316:T10)  [unwired: 4 in, 1 out]
        n225 = local write "自动切换量程"(w314) -> ()
        n226 = call <vilib>:"Close Config Data.vi"("error in (no error)"=w315, "refnum"=w316) -> ()  [unwired: 8 in, 2 out]
      }
      event "校准配置": Value Change {
        n227 = event-data() -> ()  [unwired: 1 in, 6 out]
        n228 = property on="窗格" class="Pane"("Origin"=T9 {"Horizontal"=0, "Vertical"=1300} ("原点")) -> ()  [unwired: 2 in, 2 out]
        n229 = call <vilib>:"Application Directory.vi"() -> ("Application Directory"=w385:path)
        n230 = Build Path(base path=w385, name or relative path="data\\Set.ini" ("名称或相对路径")) -> (appended path=w383:path)
        n231 = call <vilib>:"Open Config Data.vi"("configuration file path"=w383) -> ("error out"=w353:errorcluster, "refnum"=w354:T10)  [unwired: 8 in, 1 out]
        n232 = call-poly <vilib>:"Read Key.vi"("section"="CODMn模型选择" ("key"), "error in (no error)"=w353, "key"="线性和多项式", "refnum"=w354) -> ("error out"=w349:errorcluster, "value"=w352:i32, "refnum out"=w350:T10)  [unwired: 4 in, 1 out]
        n233 = local write "模型"(w352) -> ()
        n234 = call-poly <vilib>:"Read Key.vi"("section"="标线选择", "error in (no error)"=w349, "key"="选用水样", "refnum"=w350) -> ("error out"=w347:errorcluster, "value"=w351:i32, "refnum out"=w348:T10)  [unwired: 4 in, 1 out]
        n235 = local write "选用水样"(w351) -> ()
        n236 = local read "量程选择"() -> (w360:enum16{"低量程", "高量程"})
        n237 = case shown="0, 默认" w351 {
          tunnel: ["葡萄糖标线" ("section") "草酸钠标线" ("section")] -> w359
          frame 0, Default {
          }
          frame 1 {
          }
        }
        n238 = case shown="\"高量程\"" w360 {
          tunnel: ["低量程" "高量程"] -> w358
          frame "低量程", Default {
          }
          frame "高量程" {
          }
        }
        n239 = Concatenate Strings(w359, w358) -> (w357:string)
        n240 = call-poly <vilib>:"Read Key.vi"("section"=w357, "error in (no error)"=w347, "key"="浓度1", "refnum"=w348) -> ("error out"=w389:errorcluster, "value"=w387:dbl, "refnum out"=w388:T10)  [unwired: 4 in, 1 out]
        n241 = local write "浓度1"(w387) -> ()
        n242 = call-poly <vilib>:"Read Key.vi"("section"=w357, "error in (no error)"=w389, "key"="浓度2", "refnum"=w388) -> ("error out"=w403:errorcluster, "value"=w390:dbl, "refnum out"=w402:T10)  [unwired: 4 in, 1 out]
        n243 = local write "浓度2"(w390) -> ()
        n244 = call-poly <vilib>:"Read Key.vi"("section"=w357, "error in (no error)"=w403, "key"="浓度3", "refnum"=w402) -> ("error out"=w404:errorcluster, "value"=w392:dbl, "refnum out"=w401:T10)  [unwired: 4 in, 1 out]
        n245 = local write "浓度3"(w392) -> ()
        n246 = call-poly <vilib>:"Read Key.vi"("section"=w357, "error in (no error)"=w404, "key"="泵滴定数1", "refnum"=w401) -> ("error out"=w405:errorcluster, "value"=w394:dbl, "refnum out"=w400:T10)  [unwired: 4 in, 1 out]
        n247 = local write "泵滴定数1"(w394) -> ()
        n248 = call-poly <vilib>:"Read Key.vi"("section"=w357, "error in (no error)"=w405, "key"="泵滴定数2", "refnum"=w400) -> ("error out"=w399:errorcluster, "value"=w397:dbl, "refnum out"=w406:T10)  [unwired: 4 in, 1 out]
        n249 = local write "泵滴定数2"(w397) -> ()
        n250 = call-poly <vilib>:"Read Key.vi"("section"=w357, "error in (no error)"=w399, "key"="泵滴定数3", "refnum"=w406) -> ("error out"=w411:errorcluster, "value"=w410:dbl, "refnum out"=w407:T10)  [unwired: 4 in, 1 out]
        n251 = local write "泵滴定数3"(w410) -> ()
        n252 = call-poly <vilib>:"Read Key.vi"("section"=w357, "error in (no error)"=w411, "key"="浓度4", "refnum"=w407) -> ("error out"=w412:errorcluster, "value"=w340:dbl, "refnum out"=w408:T10)  [unwired: 4 in, 1 out]
        n253 = local write "浓度4"(w340) -> ()
        n254 = call-poly <vilib>:"Read Key.vi"("section"=w357, "error in (no error)"=w412, "key"="浓度5", "refnum"=w408) -> ("error out"=w345:errorcluster, "value"=w339:dbl, "refnum out"=w346:T10)  [unwired: 4 in, 1 out]
        n255 = local write "浓度5"(w339) -> ()
        n256 = call-poly <vilib>:"Read Key.vi"("section"=w357, "error in (no error)"=w345, "key"="泵滴定数4", "refnum"=w346) -> ("error out"=w413:errorcluster, "value"=w338:dbl, "refnum out"=w409:T10)  [unwired: 4 in, 1 out]
        n257 = local write "泵滴定数4"(w338) -> ()
        n258 = call-poly <vilib>:"Read Key.vi"("section"=w357, "error in (no error)"=w413, "key"="泵滴定数5", "refnum"=w409) -> ("error out"=w343:errorcluster, "value"=w337:dbl, "refnum out"=w344:T10)  [unwired: 4 in, 1 out]
        n259 = local write "泵滴定数5"(w337) -> ()
        n260 = call-poly <vilib>:"Read Key.vi"("section"=w357, "error in (no error)"=w343, "key"="当前选用的校准", "refnum"=w344) -> ("error out"=w379:errorcluster, "value"=w381:i32, "refnum out"=w380:T10)  [unwired: 4 in, 1 out]
        n261 = local write "当前校准"(w381) -> ()
        n262 = call-poly <vilib>:"Read Key.vi"("section"=w357, "error in (no error)"=w379, "key"="启用1", "refnum"=w380) -> ("error out"=w376:errorcluster, "value"=w365:bool, "refnum out"=w377:T10)  [unwired: 4 in, 1 out]
        n263 = local write "启用1"(w365) -> ()
        n264 = call-poly <vilib>:"Read Key.vi"("section"=w357, "error in (no error)"=w376, "key"="启用2", "refnum"=w377) -> ("error out"=w374:errorcluster, "value"=w364:bool, "refnum out"=w375:T10)  [unwired: 4 in, 1 out]
        n265 = local write "启用2"(w364) -> ()
        n266 = call-poly <vilib>:"Read Key.vi"("section"=w357, "error in (no error)"=w374, "key"="启用3", "refnum"=w375) -> ("error out"=w372:errorcluster, "value"=w363:bool, "refnum out"=w373:T10)  [unwired: 4 in, 1 out]
        n267 = local write "启用3"(w363) -> ()
        n268 = call-poly <vilib>:"Read Key.vi"("section"=w357, "error in (no error)"=w372, "key"="启用4", "refnum"=w373) -> ("error out"=w370:errorcluster, "value"=w336:bool, "refnum out"=w371:T10)  [unwired: 4 in, 1 out]
        n269 = local write "启用4"(w336) -> ()
        n270 = call-poly <vilib>:"Read Key.vi"("section"=w357, "error in (no error)"=w370, "key"="启用5", "refnum"=w371) -> ("error out"=w341:errorcluster, "value"=w335:bool, "refnum out"=w342:T10)  [unwired: 4 in, 1 out]
        n271 = local write "启用5"(w335) -> ()
        n272 = call <vilib>:"Close Config Data.vi"("error in (no error)"=w341, "refnum"=w342) -> ()  [unwired: 8 in, 2 out]
      }
      event "选用水样": Value Change {
        (unwired) "浓度6" ("key")
        n273 = event-data() -> ()  [unwired: 1 in, 6 out]
        n274 = property on="窗格" class="Pane"("Origin"=T9 {"Horizontal"=0, "Vertical"=1300} ("原点")) -> ()  [unwired: 2 in, 2 out]
        n275 = local read "量程选择"() -> (w436:enum16{"低量程", "高量程"})
        n276 = case shown="\"高量程\"" w436 {
          tunnel: ["低量程" "高量程"] -> w437
          frame "低量程", Default {
          }
          frame "高量程" {
          }
        }
        n277 = case shown="\"葡萄糖\", 默认" "选用水样" {
          tunnel: ["葡萄糖标线" ("section") "草酸钠标线" ("section")] -> w438
          frame "葡萄糖", Default {
          }
          frame "草酸钠" {
          }
        }
        n278 = call <vilib>:"Application Directory.vi"() -> ("Application Directory"=w462:path)
        n279 = Build Path(base path=w462, name or relative path="data\\Set.ini" ("名称或相对路径")) -> (appended path=w460:path)
        n280 = call <vilib>:"Open Config Data.vi"("configuration file path"=w460) -> ("error out"=w463:errorcluster, "refnum"=w464:T10)  [unwired: 8 in, 1 out]
        n281 = Concatenate Strings(w438, w437) -> (w435:string)
        n282 = call-poly <vilib>:"Read Key.vi"("section"=w435, "error in (no error)"=w463, "key"="浓度1", "refnum"=w464) -> ("error out"=w468:errorcluster, "value"=w466:dbl, "refnum out"=w467:T10)  [unwired: 4 in, 1 out]
        n283 = local write "浓度1"(w466) -> ()
        n284 = call-poly <vilib>:"Read Key.vi"("section"=w435, "error in (no error)"=w468, "key"="浓度2", "refnum"=w467) -> ("error out"=w482:errorcluster, "value"=w469:dbl, "refnum out"=w481:T10)  [unwired: 4 in, 1 out]
        n285 = local write "浓度2"(w469) -> ()
        n286 = call-poly <vilib>:"Read Key.vi"("section"=w435, "error in (no error)"=w482, "key"="浓度3", "refnum"=w481) -> ("error out"=w483:errorcluster, "value"=w471:dbl, "refnum out"=w480:T10)  [unwired: 4 in, 1 out]
        n287 = local write "浓度3"(w471) -> ()
        n288 = call-poly <vilib>:"Read Key.vi"("section"=w435, "error in (no error)"=w483, "key"="泵滴定数1", "refnum"=w480) -> ("error out"=w484:errorcluster, "value"=w473:dbl, "refnum out"=w479:T10)  [unwired: 4 in, 1 out]
        n289 = local write "泵滴定数1"(w473) -> ()
        n290 = call-poly <vilib>:"Read Key.vi"("section"=w435, "error in (no error)"=w484, "key"="泵滴定数2", "refnum"=w479) -> ("error out"=w478:errorcluster, "value"=w476:dbl, "refnum out"=w485:T10)  [unwired: 4 in, 1 out]
        n291 = local write "泵滴定数2"(w476) -> ()
        n292 = call-poly <vilib>:"Read Key.vi"("section"=w435, "error in (no error)"=w478, "key"="泵滴定数3", "refnum"=w485) -> ("error out"=w490:errorcluster, "value"=w489:dbl, "refnum out"=w486:T10)  [unwired: 4 in, 1 out]
        n293 = local write "泵滴定数3"(w489) -> ()
        n294 = call-poly <vilib>:"Read Key.vi"("section"=w435, "error in (no error)"=w490, "key"="浓度4", "refnum"=w486) -> ("error out"=w491:errorcluster, "value"=w430:dbl, "refnum out"=w487:T10)  [unwired: 4 in, 1 out]
        n295 = local write "浓度4"(w430) -> ()
        n296 = call-poly <vilib>:"Read Key.vi"("section"=w435, "error in (no error)"=w491, "key"="浓度5", "refnum"=w487) -> ("error out"=w433:errorcluster, "value"=w429:dbl, "refnum out"=w434:T10)  [unwired: 4 in, 1 out]
        n297 = local write "浓度5"(w429) -> ()
        n298 = call-poly <vilib>:"Read Key.vi"("section"=w435, "error in (no error)"=w433, "key"="泵滴定数4", "refnum"=w434) -> ("error out"=w492:errorcluster, "value"=w428:dbl, "refnum out"=w488:T10)  [unwired: 4 in, 1 out]
        n299 = local write "泵滴定数4"(w428) -> ()
        n300 = call-poly <vilib>:"Read Key.vi"("section"=w435, "error in (no error)"=w492, "key"="泵滴定数5", "refnum"=w488) -> ("error out"=w431:errorcluster, "value"=w427:dbl, "refnum out"=w432:T10)  [unwired: 4 in, 1 out]
        n301 = local write "泵滴定数5"(w427) -> ()
        n302 = call-poly <vilib>:"Read Key.vi"("section"=w435, "error in (no error)"=w431, "key"="当前选用的校准", "refnum"=w432) -> ("error out"=w456:errorcluster, "value"=w458:i32, "refnum out"=w457:T10)  [unwired: 4 in, 1 out]
        n303 = local write "当前校准"(w458) -> ()
        n304 = call-poly <vilib>:"Read Key.vi"("section"=w435, "error in (no error)"=w456, "key"="启用1", "refnum"=w457) -> ("error out"=w453:errorcluster, "value"=w442:bool, "refnum out"=w454:T10)  [unwired: 4 in, 1 out]
        n305 = local write "启用1"(w442) -> ()
        n306 = call-poly <vilib>:"Read Key.vi"("section"=w435, "error in (no error)"=w453, "key"="启用2", "refnum"=w454) -> ("error out"=w451:errorcluster, "value"=w441:bool, "refnum out"=w452:T10)  [unwired: 4 in, 1 out]
        n307 = local write "启用2"(w441) -> ()
        n308 = call-poly <vilib>:"Read Key.vi"("section"=w435, "error in (no error)"=w451, "key"="启用3", "refnum"=w452) -> ("error out"=w449:errorcluster, "value"=w440:bool, "refnum out"=w450:T10)  [unwired: 4 in, 1 out]
        n309 = local write "启用3"(w440) -> ()
        n310 = call-poly <vilib>:"Read Key.vi"("section"=w435, "error in (no error)"=w449, "key"="启用4", "refnum"=w450) -> ("error out"=w447:errorcluster, "value"=w424:bool, "refnum out"=w448:T10)  [unwired: 4 in, 1 out]
        n311 = local write "启用4"(w424) -> ()
        n312 = call-poly <vilib>:"Read Key.vi"("section"=w435, "error in (no error)"=w447, "key"="启用5", "refnum"=w448) -> ("error out"=w425:errorcluster, "value"=w423:bool, "refnum out"=w426:T10)  [unwired: 4 in, 1 out]
        n313 = local write "启用5"(w423) -> ()
        n314 = call <vilib>:"Close Config Data.vi"("error in (no error)"=w425, "refnum"=w426) -> ()  [unwired: 8 in, 2 out]
      }
      event "量程选择": Value Change {
        n315 = event-data() -> ()  [unwired: 1 in, 6 out]
        n316 = property on="窗格" class="Pane"("Origin"=T9 {"Horizontal"=0, "Vertical"=1300} ("原点")) -> ()  [unwired: 2 in, 2 out]
        n317 = local read "选用水样"() -> (w518:enum16{"葡萄糖", "草酸钠"})
        n318 = case shown="\"葡萄糖\", 默认" w518 {
          tunnel: ["葡萄糖标线" ("section") "草酸钠标线" ("section")] -> w517
          frame "葡萄糖", Default {
          }
          frame "草酸钠" {
          }
        }
        n319 = case shown="\"高量程\"" "量程选择" {
          tunnel: ["低量程" "高量程"] -> w514
          frame "低量程", Default {
          }
          frame "高量程" {
          }
        }
        n320 = call <vilib>:"Application Directory.vi"() -> ("Application Directory"=w541:path)
        n321 = Build Path(base path=w541, name or relative path="data\\Set.ini" ("名称或相对路径")) -> (appended path=w539:path)
        n322 = call <vilib>:"Open Config Data.vi"("configuration file path"=w539) -> ("error out"=w542:errorcluster, "refnum"=w543:T10)  [unwired: 8 in, 1 out]
        n323 = Concatenate Strings(w517, w514) -> (w516:string)
        n324 = call-poly <vilib>:"Read Key.vi"("section"=w516, "error in (no error)"=w542, "key"="浓度1", "refnum"=w543) -> ("error out"=w547:errorcluster, "value"=w545:dbl, "refnum out"=w546:T10)  [unwired: 4 in, 1 out]
        n325 = local write "浓度1"(w545) -> ()
        n326 = call-poly <vilib>:"Read Key.vi"("section"=w516, "error in (no error)"=w547, "key"="浓度2", "refnum"=w546) -> ("error out"=w561:errorcluster, "value"=w548:dbl, "refnum out"=w560:T10)  [unwired: 4 in, 1 out]
        n327 = local write "浓度2"(w548) -> ()
        n328 = call-poly <vilib>:"Read Key.vi"("section"=w516, "error in (no error)"=w561, "key"="浓度3", "refnum"=w560) -> ("error out"=w562:errorcluster, "value"=w550:dbl, "refnum out"=w559:T10)  [unwired: 4 in, 1 out]
        n329 = local write "浓度3"(w550) -> ()
        n330 = call-poly <vilib>:"Read Key.vi"("section"=w516, "error in (no error)"=w562, "key"="泵滴定数1", "refnum"=w559) -> ("error out"=w563:errorcluster, "value"=w552:dbl, "refnum out"=w558:T10)  [unwired: 4 in, 1 out]
        n331 = local write "泵滴定数1"(w552) -> ()
        n332 = call-poly <vilib>:"Read Key.vi"("section"=w516, "error in (no error)"=w563, "key"="泵滴定数2", "refnum"=w558) -> ("error out"=w557:errorcluster, "value"=w555:dbl, "refnum out"=w564:T10)  [unwired: 4 in, 1 out]
        n333 = local write "泵滴定数2"(w555) -> ()
        n334 = call-poly <vilib>:"Read Key.vi"("section"=w516, "error in (no error)"=w557, "key"="泵滴定数3", "refnum"=w564) -> ("error out"=w569:errorcluster, "value"=w568:dbl, "refnum out"=w565:T10)  [unwired: 4 in, 1 out]
        n335 = local write "泵滴定数3"(w568) -> ()
        n336 = call-poly <vilib>:"Read Key.vi"("section"=w516, "error in (no error)"=w569, "key"="浓度4", "refnum"=w565) -> ("error out"=w570:errorcluster, "value"=w505:dbl, "refnum out"=w566:T10)  [unwired: 4 in, 1 out]
        n337 = local write "浓度4"(w505) -> ()
        n338 = call-poly <vilib>:"Read Key.vi"("section"=w516, "error in (no error)"=w570, "key"="浓度5", "refnum"=w566) -> ("error out"=w512:errorcluster, "value"=w504:dbl, "refnum out"=w513:T10)  [unwired: 4 in, 1 out]
        n339 = local write "浓度5"(w504) -> ()
        n340 = call-poly <vilib>:"Read Key.vi"("section"=w516, "error in (no error)"=w512, "key"="泵滴定数4", "refnum"=w513) -> ("error out"=w571:errorcluster, "value"=w503:dbl, "refnum out"=w567:T10)  [unwired: 4 in, 1 out]
        n341 = local write "泵滴定数4"(w503) -> ()
        n342 = call-poly <vilib>:"Read Key.vi"("section"=w516, "error in (no error)"=w571, "key"="泵滴定数5", "refnum"=w567) -> ("error out"=w510:errorcluster, "value"=w502:dbl, "refnum out"=w511:T10)  [unwired: 4 in, 1 out]
        n343 = local write "泵滴定数5"(w502) -> ()
        n344 = call-poly <vilib>:"Read Key.vi"("section"=w516, "error in (no error)"=w510, "key"="当前选用的校准", "refnum"=w511) -> ("error out"=w535:errorcluster, "value"=w537:i32, "refnum out"=w536:T10)  [unwired: 4 in, 1 out]
        n345 = local write "当前校准"(w537) -> ()
        n346 = call-poly <vilib>:"Read Key.vi"("section"=w516, "error in (no error)"=w535, "key"="启用1", "refnum"=w536) -> ("error out"=w532:errorcluster, "value"=w521:bool, "refnum out"=w533:T10)  [unwired: 4 in, 1 out]
        n347 = local write "启用1"(w521) -> ()
        n348 = call-poly <vilib>:"Read Key.vi"("section"=w516, "error in (no error)"=w532, "key"="启用2", "refnum"=w533) -> ("error out"=w530:errorcluster, "value"=w520:bool, "refnum out"=w531:T10)  [unwired: 4 in, 1 out]
        n349 = local write "启用2"(w520) -> ()
        n350 = call-poly <vilib>:"Read Key.vi"("section"=w516, "error in (no error)"=w530, "key"="启用3", "refnum"=w531) -> ("error out"=w528:errorcluster, "value"=w519:bool, "refnum out"=w529:T10)  [unwired: 4 in, 1 out]
        n351 = local write "启用3"(w519) -> ()
        n352 = call-poly <vilib>:"Read Key.vi"("section"=w516, "error in (no error)"=w528, "key"="启用4", "refnum"=w529) -> ("error out"=w526:errorcluster, "value"=w507:bool, "refnum out"=w527:T10)  [unwired: 4 in, 1 out]
        n353 = local write "启用4"(w507) -> ()
        n354 = call-poly <vilib>:"Read Key.vi"("section"=w516, "error in (no error)"=w526, "key"="启用5", "refnum"=w527) -> ("error out"=w508:errorcluster, "value"=w506:bool, "refnum out"=w509:T10)  [unwired: 4 in, 1 out]
        n355 = local write "启用5"(w506) -> ()
        n356 = call <vilib>:"Close Config Data.vi"("error in (no error)"=w508, "refnum"=w509) -> ()  [unwired: 8 in, 2 out]
      }
      event "周期设置": Value Change {
        n357 = event-data() -> ()  [unwired: 1 in, 6 out]
        n358 = disable-structure shown="禁用" {
          disable-tunnel: [w584 _] -> _
          frame Disabled {
            n359 = call "请输入管理员密码"() -> ("确定"=w584:bool)  [unwired: 17 in, 2 out]
          }
          frame Enabled {
          }
        }
        n360 = call "数字密码键盘.vi"() -> ("NewNumber"=w581:sgl)  [unwired: 1 in]
        n361 = Equal?(x=w581, y=8.0) -> (x = y?=w582:bool)
        n362 = case shown="真" w582 {
          frame False {
            n363 = call "窗口弹出对话框(子VI).vi"("消息"="密码错误") -> ()  [unwired: 10 in, 1 out]
          }
          frame True {
            n364 = call "窗口弹出对话框(子VI).vi"("消息"="登录成功") -> ("true"=w586:bool)  [unwired: 10 in]
            n365 = case shown="真" w586 {
              frame False {
              }
              frame True {
                n366 = property on="窗格" class="Pane"("Origin"=T9 {"Horizontal"=0, "Vertical"=1950} ("原点")) -> ()  [unwired: 2 in, 2 out]
              }
            }
          }
        }
      }
      event "返回": Value Change {
        (unwired) "泵滴定数6" ("key")
        w602 = "CODMn" ("section")
        n367 = event-data() -> ()  [unwired: 1 in, 6 out]
        n368 = property on="窗格" class="Pane"("Origin"=T9 {"Horizontal"=0, "Vertical"=0} ("原点")) -> ()  [unwired: 2 in, 2 out]
        n369 = call <vilib>:"Application Directory.vi"() -> ("Application Directory"=w655:path)
        n370 = Build Path(base path=w655, name or relative path="data\\Set.ini" ("名称或相对路径")) -> (appended path=w653:path)
        n371 = local write "读取KB值"(FALSE ("读取KB值")) -> ()
        n372 = call <vilib>:"Open Config Data.vi"("configuration file path"=w653) -> ("error out"=w651:errorcluster, "refnum"=w652:T10)  [unwired: 8 in, 1 out]
        n373 = local read "浓度1"() -> (w649:dbl)
        n374 = local read "浓度2"() -> (w633:dbl)
        n375 = call-poly <vilib>:"Write Key.vi"("section"=w602, "error in (no error)"=w651, "value"=w649, "key"="浓度1", "refnum"=w652) -> ("error out"=w648:errorcluster, "refnum out"=w647:T10)  [unwired: 4 in, 1 out]
        n376 = local read "浓度3"() -> (w629:dbl)
        n377 = call-poly <vilib>:"Write Key.vi"("section"=w602, "error in (no error)"=w648, "value"=w633, "key"="浓度2", "refnum"=w647) -> ("error out"=w646:errorcluster, "refnum out"=w645:T10)  [unwired: 4 in, 1 out]
        n378 = local read "泵滴定数1"() -> (w627:dbl)
        n379 = call-poly <vilib>:"Write Key.vi"("section"=w602, "error in (no error)"=w646, "value"=w629, "key"="浓度3", "refnum"=w645) -> ("error out"=w644:errorcluster, "refnum out"=w643:T10)  [unwired: 4 in, 1 out]
        n380 = call-poly <vilib>:"Write Key.vi"("section"=w602, "error in (no error)"=w644, "value"=w627, "key"="泵滴定数1", "refnum"=w643) -> ("error out"=w642:errorcluster, "refnum out"=w641:T10)  [unwired: 4 in, 1 out]
        n381 = local read "泵滴定数2"() -> (w625:dbl)
        n382 = call-poly <vilib>:"Write Key.vi"("section"=w602, "error in (no error)"=w642, "value"=w625, "key"="泵滴定数2", "refnum"=w641) -> ("error out"=w640:errorcluster, "refnum out"=w639:T10)  [unwired: 4 in, 1 out]
        n383 = local read "泵滴定数3"() -> (w623:dbl)
        n384 = local read "浓度4"() -> (w590:dbl)
        n385 = call-poly <vilib>:"Write Key.vi"("section"=w602, "error in (no error)"=w640, "value"=w623, "key"="泵滴定数3", "refnum"=w639) -> ("error out"=w638:errorcluster, "refnum out"=w637:T10)  [unwired: 4 in, 1 out]
        n386 = call-poly <vilib>:"Write Key.vi"("section"=w602, "error in (no error)"=w638, "value"=w590, "key"="浓度4", "refnum"=w637) -> ("error out"=w631:errorcluster, "refnum out"=w632:T10)  [unwired: 4 in, 1 out]
        n387 = local read "浓度5"() -> (w589:dbl)
        n388 = call-poly <vilib>:"Write Key.vi"("section"=w602, "error in (no error)"=w631, "value"=w589, "key"="浓度5", "refnum"=w632) -> ("error out"=w599:errorcluster, "refnum out"=w600:T10)  [unwired: 4 in, 1 out]
        n389 = local read "泵滴定数4"() -> (w591:dbl)
        n390 = call-poly <vilib>:"Write Key.vi"("section"=w602, "error in (no error)"=w599, "value"=w591, "key"="泵滴定数4", "refnum"=w600) -> ("error out"=w636:errorcluster, "refnum out"=w635:T10)  [unwired: 4 in, 1 out]
        n391 = local read "泵滴定数5"() -> (w592:dbl)
        n392 = call-poly <vilib>:"Write Key.vi"("section"=w602, "error in (no error)"=w636, "value"=w592, "key"="泵滴定数5", "refnum"=w635) -> ("error out"=w597:errorcluster, "refnum out"=w598:T10)  [unwired: 4 in, 1 out]
        n393 = local read "启用1"() -> (w611:bool)
        n394 = call-poly <vilib>:"Write Key.vi"("section"=w602, "error in (no error)"=w597, "value"=w611, "key"="启用1", "refnum"=w598) -> ("error out"=w607:errorcluster, "refnum out"=w610:T10)  [unwired: 4 in, 1 out]
        n395 = local read "启用2"() -> (w608:bool)
        n396 = call-poly <vilib>:"Write Key.vi"("section"=w602, "error in (no error)"=w607, "value"=w608, "key"="启用2", "refnum"=w610) -> ("error out"=w618:errorcluster, "refnum out"=w617:T10)  [unwired: 4 in, 1 out]
        n397 = local read "启用3"() -> (w606:bool)
        n398 = call-poly <vilib>:"Write Key.vi"("section"=w602, "error in (no error)"=w618, "value"=w606, "key"="启用3", "refnum"=w617) -> ("error out"=w616:errorcluster, "refnum out"=w615:T10)  [unwired: 4 in, 1 out]
        n399 = local read "启用4"() -> (w594:bool)
        n400 = call-poly <vilib>:"Write Key.vi"("section"=w602, "error in (no error)"=w616, "value"=w594, "key"="启用4", "refnum"=w615) -> ("error out"=w614:errorcluster, "refnum out"=w613:T10)  [unwired: 4 in, 1 out]
        n401 = local read "启用5"() -> (w593:bool)
        n402 = call-poly <vilib>:"Write Key.vi"("section"=w602, "error in (no error)"=w614, "value"=w593, "key"="启用5", "refnum"=w613) -> ("error out"=w595:errorcluster, "refnum out"=w596:T10)  [unwired: 4 in, 1 out]
        n403 = call <vilib>:"Close Config Data.vi"("error in (no error)"=w595, "refnum"=w596) -> ()  [unwired: 8 in, 2 out]
      }
      event "关闭", "关闭 2", "关闭 3": Value Change {
        n404 = event-data() -> ()  [unwired: 1 in, 6 out]
        n405 = property on="窗格" class="Pane"("Origin"=T9 {"Horizontal"=0, "Vertical"=0} ("原点")) -> ()  [unwired: 2 in, 2 out]
      }
      event Timeout; Application Instance Close {
        n406 = event-data() -> ()  [unwired: 1 in, 3 out]
        n407 = call-dynamic "Close Session.vi"("error in (no error)"=w658, "MB_Serial session"=w659) -> ()  [unwired: 9 in, 1 out]
      }
      event "时间校准": Value Change {
        n408 = event-data() -> ()  [unwired: 1 in, 6 out]
        n409 = flat-sequence {
          tunnel: w660 -> [w665]
          frame #0 {
            n410 = Get Date/Time In Seconds() -> (seconds since 1Jan1904=w670:timestamp)
            n411 = Build Array(w670) -> (w669:timestamp[])
            n412 = call "DateToHex.vi"("DATE"=w669) -> ("数组"=w663:u16[])  [unwired: 10 in]
            n413 = Insert Into Array(array=u16[] [1] ("values"), index=1 ("索引"), new element=w663) -> (w661:u16[])
            n414 = Bundle By Name(cluster=cluster{"starting address":u16, "values":u16[]} {"starting address"=0, "values"=[]}, "starting address"=u16 4612, "values"=w661) -> (w666:cluster{"starting address":u16, "values":u16[]})
            n415 = Enqueue Element(queue=w665, element=w666) -> ()  [unwired: 2 in, 3 out]
          }
          frame #1 {
            n416 = local write "枚举"(enum16{"读取数据", "写入数据", "读取写入DATABASE", "读取参数"}."写入数据" ("枚举")) -> ()
          }
        }
      }
      event "故障清除": Value Change {
        n417 = event-data() -> ()  [unwired: 1 in, 6 out]
        n418 = local write "枚举"(enum16{"读取数据", "写入数据", "读取写入DATABASE", "读取参数"}."写入数据" ("枚举")) -> ()
        n419 = Bundle By Name(cluster=cluster{"starting address":u16, "values":u16[]} {"starting address"=0, "values"=[]}, "starting address"=u16 4611, "values"=u16[] [1]) -> (w675:cluster{"starting address":u16, "values":u16[]})
        n420 = Enqueue Element(queue=w674, element=w675) -> ()  [unwired: 2 in, 3 out]
      }
      event "定时启动": Value Change {
        n421 = event-data() -> ()  [unwired: 1 in, 6 out]
        n422 = call "COD定时启动对话框.vi"() -> ("设置值"=→"定时时间":dbl, "确定输出"=w678:bool)  [unwired: 10 in]
        n423 = local write "定时启动"(w678) -> ()
      }
      event "校准1", "校准2", "校准3", "校准4", "校准5": Value Change {
        n424 = event-data() -> ()  [unwired: 1 in, 6 out]
        n425 = flat-sequence {
          tunnel: w682 -> [w687]
          tunnel: [w686] -> w681
          tunnel: [w685] -> w680
          tunnel: w681 -> [w720]
          tunnel: w680 -> [w719]
          frame #0 {
            n426 = Build Array("校准1", "校准2", "校准3", "校准4", "校准5") -> (w688:bool[])
            n427 = for {
              tunnel: w688 -> [w702] mode=indexing
              tunnel: w687 -> [w698]
              tunnel: [w694] -> w686
              tunnel: [w693] -> w685
              i -> [w692]
              n428 = case shown="4" w692 {
                tunnel: ["浓度1" "浓度2" "浓度3" "浓度4" "浓度5"] -> w697
                frame 0, Default {
                }
                frame 1 {
                }
                frame 2 {
                }
                frame 3 {
                }
                frame 4 {
                }
              }
              n429 = Multiply(x=w697, y=100.0) -> (x*y=w695:dbl)
              n430 = Insert Into Array(array=u16[] [] ("values"), index=0 ("索引"), new element=w695) -> (w699:u16[])
              n431 = case shown="真" w702 {
                tunnel: w699 -> [_ w714]
                tunnel: w698 -> [w708 w713]
                tunnel: [w708 w712] -> w694
                tunnel: [_ w711] -> w693
                tunnel: w692 -> [_ w710]
                frame False {
                }
                frame True {
                  n432 = Increment(x=w710) -> (x+1=→"当前校准":i32)
                  n433 = Bundle By Name(cluster=cluster{"starting address":u16, "values":u16[]} {"starting address"=4272, "values"=[]}, "starting address"=u16 4274, "values"=w714) -> (w716:cluster{"starting address":u16, "values":u16[]})
                  n434 = Enqueue Element(queue=w713, element=w716) -> (queue out=w712:refnum<queue>, error out=w711:errorcluster)  [unwired: 2 in, 1 out]
                }
              }
            }
          }
          frame #1 {
            n435 = local read "当前校准"() -> (w725:i32)
            n436 = case shown="5" w725 {
              tunnel: [w731 w732 w733 w734 w735] -> w724
              frame 1, Default {
                n437 = local read "浓度1"() -> (w731:dbl)
              }
              frame 2 {
                n438 = local read "浓度2"() -> (w732:dbl)
              }
              frame 3 {
                n439 = local read "浓度3"() -> (w733:dbl)
              }
              frame 4 {
                n440 = local read "浓度4"() -> (w734:dbl)
              }
              frame 5 {
                n441 = local read "浓度5"() -> (w735:dbl)
              }
            }
            n442 = Not Equal To 0?(x=w724) -> (x != 0?=w723:bool)
            n443 = case shown="真" w723 {
              tunnel: [u16 8 ("address") u16 9 ("address")] -> w728
              tunnel: ["校零" ("测量模式") "校标" ("测量模式")] -> w718
              frame False {
              }
              frame True {
              }
            }
            n444 = global write "COD测量模式全局.vi" "测量模式"(w718) -> ()
            n445 = Insert Into Array(array=u16[] [] ("values"), index=0 ("索引"), new element=w728) -> (w722:u16[])
            n446 = Bundle By Name(cluster=cluster{"starting address":u16, "values":u16[]} {"starting address"=0, "values"=[]}, "starting address"=u16 4608 ("address"), "values"=w722) -> (w730:cluster{"starting address":u16, "values":u16[]})
            n447 = Enqueue Element(queue=w720, element=w730, error in (no error)=w719) -> ()  [unwired: 1 in, 3 out]
          }
          frame #2 {
            n448 = local write "枚举"(enum16{"读取数据", "写入数据", "读取写入DATABASE", "读取参数"}."写入数据" ("枚举")) -> ()
            n449 = call <vilib>:"Application Directory.vi"() -> ("Application Directory"=w747:path)
            n450 = Build Path(base path=w747, name or relative path="data\\Set.ini" ("名称或相对路径")) -> (appended path=w749:path)
            n451 = local read "当前校准"() -> (w742:i32)
            n452 = call <vilib>:"Open Config Data.vi"("configuration file path"=w749) -> ("error out"=w745:errorcluster, "refnum"=w746:T10)  [unwired: 8 in, 1 out]
            n453 = call-poly <vilib>:"Write Key.vi"("section"="CODMn", "error in (no error)"=w745, "value"=w742, "key"="当前选用的校准" ("section"), "refnum"=w746) -> ("error out"=w740:errorcluster, "refnum out"=w741:T10)  [unwired: 4 in, 1 out]
            n454 = call <vilib>:"Close Config Data.vi"("error in (no error)"=w740, "refnum"=w741) -> ()  [unwired: 8 in, 2 out]
          }
        }
      }
      event "自动切换量程": Value Change {
        n455 = event-data() -> ()  [unwired: 1 in, 6 out]
        n456 = call <vilib>:"Application Directory.vi"() -> ("Application Directory"=w760:path)
        n457 = Build Path(base path=w760, name or relative path="data\\Set.ini" ("名称或相对路径")) -> (appended path=w758:path)
        n458 = local read "自动切换量程"() -> (w753:bool)
        n459 = call <vilib>:"Open Config Data.vi"("configuration file path"=w758) -> ("error out"=w756:errorcluster, "refnum"=w757:T10)  [unwired: 8 in, 1 out]
        n460 = call-poly <vilib>:"Write Key.vi"("section"="CODMn是否切换量程" ("key"), "error in (no error)"=w756, "value"=w753, "key"="自动切换量程", "refnum"=w757) -> ("error out"=w751:errorcluster, "refnum out"=w752:T10)  [unwired: 4 in, 1 out]
        n461 = call <vilib>:"Close Config Data.vi"("error in (no error)"=w751, "refnum"=w752) -> ()  [unwired: 8 in, 2 out]
      }
      event "模型": Value Change {
        n462 = event-data() -> ()  [unwired: 1 in, 6 out]
        n463 = call <vilib>:"Application Directory.vi"() -> ("Application Directory"=w770:path)
        n464 = Build Path(base path=w770, name or relative path="data\\Set.ini" ("名称或相对路径")) -> (appended path=w768:path)
        n465 = call <vilib>:"Open Config Data.vi"("configuration file path"=w768) -> ("error out"=w766:errorcluster, "refnum"=w767:T10)  [unwired: 8 in, 1 out]
        n466 = local read "模型"() -> (w761:enum32{"线性", "多项式"})
        n467 = call-poly <vilib>:"Write Key.vi"("section"="CODMn模型选择" ("key"), "error in (no error)"=w766, "value"=w761, "key"="线性和多项式", "refnum"=w767) -> ("error out"=w762:errorcluster, "refnum out"=w763:T10)  [unwired: 4 in, 1 out]
        n468 = call <vilib>:"Close Config Data.vi"("error in (no error)"=w762, "refnum"=w763) -> ()  [unwired: 8 in, 2 out]
      }
      event "浓度1", "浓度2", "浓度3", "泵滴定数1", "泵滴定数2", "泵滴定数3", "启用1", "启用2", "启用3", "浓度4", "浓度5", "泵滴定数4", "泵滴定数5", "启用4", "启用5": Value Change {
        n469 = event-data() -> ()  [unwired: 1 in, 6 out]
        n470 = local read "选用水样"() -> (w786:enum16{"葡萄糖", "草酸钠"})
        n471 = local read "量程选择"() -> (w785:enum16{"低量程", "高量程"})
        n472 = case shown="\"高量程\"" w785 {
          tunnel: ["低量程" "高量程"] -> w783
          frame "低量程", Default {
          }
          frame "高量程" {
          }
        }
        n473 = call <vilib>:"Application Directory.vi"() -> ("Application Directory"=w845:path)
        n474 = case shown="\"葡萄糖\", 默认" w786 {
          tunnel: ["葡萄糖标线" ("section") "草酸钠标线" ("section")] -> w792
          frame "葡萄糖", Default {
          }
          frame "草酸钠" {
          }
        }
        n475 = Build Path(base path=w845, name or relative path="data\\Set.ini" ("名称或相对路径")) -> (appended path=w843:path)
        n476 = call <vilib>:"Open Config Data.vi"("configuration file path"=w843) -> ("error out"=w841:errorcluster, "refnum"=w842:T10)  [unwired: 8 in, 1 out]
        n477 = local read "浓度1"() -> (w839:dbl)
        n478 = Concatenate Strings(w792, w783) -> (w784:string)
        n479 = local read "浓度2"() -> (w823:dbl)
        n480 = call-poly <vilib>:"Write Key.vi"("section"=w784, "error in (no error)"=w841, "value"=w839, "key"="浓度1", "refnum"=w842) -> ("error out"=w838:errorcluster, "refnum out"=w837:T10)  [unwired: 4 in, 1 out]
        n481 = local read "浓度3"() -> (w819:dbl)
        n482 = call-poly <vilib>:"Write Key.vi"("section"=w784, "error in (no error)"=w838, "value"=w823, "key"="浓度2", "refnum"=w837) -> ("error out"=w836:errorcluster, "refnum out"=w835:T10)  [unwired: 4 in, 1 out]
        n483 = local read "泵滴定数1"() -> (w817:dbl)
        n484 = call-poly <vilib>:"Write Key.vi"("section"=w784, "error in (no error)"=w836, "value"=w819, "key"="浓度3", "refnum"=w835) -> ("error out"=w834:errorcluster, "refnum out"=w833:T10)  [unwired: 4 in, 1 out]
        n485 = call-poly <vilib>:"Write Key.vi"("section"=w784, "error in (no error)"=w834, "value"=w817, "key"="泵滴定数1", "refnum"=w833) -> ("error out"=w832:errorcluster, "refnum out"=w831:T10)  [unwired: 4 in, 1 out]
        n486 = local read "泵滴定数2"() -> (w815:dbl)
        n487 = call-poly <vilib>:"Write Key.vi"("section"=w784, "error in (no error)"=w832, "value"=w815, "key"="泵滴定数2", "refnum"=w831) -> ("error out"=w830:errorcluster, "refnum out"=w829:T10)  [unwired: 4 in, 1 out]
        n488 = local read "泵滴定数3"() -> (w813:dbl)
        n489 = local read "浓度4"() -> (w782:dbl)
        n490 = call-poly <vilib>:"Write Key.vi"("section"=w784, "error in (no error)"=w830, "value"=w813, "key"="泵滴定数3", "refnum"=w829) -> ("error out"=w828:errorcluster, "refnum out"=w827:T10)  [unwired: 4 in, 1 out]
        n491 = local read "浓度5"() -> (w781:dbl)
        n492 = call-poly <vilib>:"Write Key.vi"("section"=w784, "error in (no error)"=w828, "value"=w782, "key"="浓度4", "refnum"=w827) -> ("error out"=w821:errorcluster, "refnum out"=w822:T10)  [unwired: 4 in, 1 out]
        n493 = call-poly <vilib>:"Write Key.vi"("section"=w784, "error in (no error)"=w821, "value"=w781, "key"="浓度5", "refnum"=w822) -> ("error out"=w779:errorcluster, "refnum out"=w780:T10)  [unwired: 4 in, 1 out]
        n494 = local read "泵滴定数4"() -> (w778:dbl)
        n495 = call-poly <vilib>:"Write Key.vi"("section"=w784, "error in (no error)"=w779, "value"=w778, "key"="泵滴定数4", "refnum"=w780) -> ("error out"=w826:errorcluster, "refnum out"=w825:T10)  [unwired: 4 in, 1 out]
        n496 = local read "泵滴定数5"() -> (w777:dbl)
        n497 = call-poly <vilib>:"Write Key.vi"("section"=w784, "error in (no error)"=w826, "value"=w777, "key"="泵滴定数5", "refnum"=w825) -> ("error out"=w775:errorcluster, "refnum out"=w776:T10)  [unwired: 4 in, 1 out]
        n498 = local read "启用1"() -> (w801:bool)
        n499 = call-poly <vilib>:"Write Key.vi"("section"=w784, "error in (no error)"=w775, "value"=w801, "key"="启用1", "refnum"=w776) -> ("error out"=w797:errorcluster, "refnum out"=w800:T10)  [unwired: 4 in, 1 out]
        n500 = local read "启用2"() -> (w798:bool)
        n501 = call-poly <vilib>:"Write Key.vi"("section"=w784, "error in (no error)"=w797, "value"=w798, "key"="启用2", "refnum"=w800) -> ("error out"=w808:errorcluster, "refnum out"=w807:T10)  [unwired: 4 in, 1 out]
        n502 = local read "启用3"() -> (w796:bool)
        n503 = call-poly <vilib>:"Write Key.vi"("section"=w784, "error in (no error)"=w808, "value"=w796, "key"="启用3", "refnum"=w807) -> ("error out"=w806:errorcluster, "refnum out"=w805:T10)  [unwired: 4 in, 1 out]
        n504 = local read "启用4"() -> (w771:bool)
        n505 = call-poly <vilib>:"Write Key.vi"("section"=w784, "error in (no error)"=w806, "value"=w771, "key"="启用4", "refnum"=w805) -> ("error out"=w804:errorcluster, "refnum out"=w803:T10)  [unwired: 4 in, 1 out]
        n506 = local read "启用5"() -> (w772:bool)
        n507 = call-poly <vilib>:"Write Key.vi"("section"=w784, "error in (no error)"=w804, "value"=w772, "key"="启用5", "refnum"=w803) -> ("error out"=w773:errorcluster, "refnum out"=w774:T10)  [unwired: 4 in, 1 out]
        n508 = local read "选用水样"() -> (w791:enum16{"葡萄糖", "草酸钠"})
        n509 = call-poly <vilib>:"Write Key.vi"("section"="标线选择", "error in (no error)"=w773, "value"=w791, "key"="选用水样", "refnum"=w774) -> ("error out"=w788:errorcluster, "refnum out"=w789:T10)  [unwired: 4 in, 1 out]
        n510 = call <vilib>:"Close Config Data.vi"("error in (no error)"=w788, "refnum"=w789) -> ()  [unwired: 8 in, 2 out]
      }
      event "读取": Value Change {
        n511 = event-data() -> ()  [unwired: 1 in, 6 out]
        n512 = local write "枚举"(enum16{"读取数据", "写入数据", "读取写入DATABASE", "读取参数"}."读取参数" ("枚举")) -> ()
        n513 = Bundle By Name(cluster=T6 {"starting address"=0, "number of holding registers"=0}, "starting address"=u16 4616, "number of holding registers"=u16 22) -> (w859:T6)
        n514 = Flush Queue(queue=w852, error in (no error)=w851) -> (queue out=w855:refnum<queue>, error out=w854:errorcluster)  [unwired: 1 out]
        n515 = Enqueue Element(queue=w855, element=w859, error in (no error)=w854) -> ()  [unwired: 1 in, 3 out]
        "读取KB值" <- TRUE
      }
      event "写入": Mouse Down {
        n516 = event-data() -> ()  [unwired: 1 in, 8 out]
        n517 = flat-sequence {
          tunnel: w860 -> [w863]
          frame #0 {
            n518 = local read "模型"() -> (w861:enum32{"线性", "多项式"})
            n519 = case shown="\"多项式\"" w861 {
              tunnel: [w875 w881] -> w865
              tunnel: w863 -> [w869 w880]
              tunnel: [w869 w880] -> w862
              frame "线性", Default {
                n520 = local read "K"() -> (w872:dbl)
                n521 = local read "b"() -> (w871:dbl)
                n522 = Build Array(w872, w871, 0.0 ("元素")) -> (w870:dbl[])
                n523 = local read "量程选择"() -> (w868:enum16{"低量程", "高量程"})
                n524 = call "浮点转CDAB整形cod.vi"("浮点数"=w870) -> ("CDAB整形输出"=w873:u16[])  [unwired: 10 in]
                n525 = case shown="\"低量程\", 默认" w868 {
                  tunnel: [u16 4626 ("starting address") u16 4632 ("starting address")] -> w867
                  frame "低量程", Default {
                  }
                  frame "高量程" {
                  }
                }
                n526 = Bundle By Name(cluster=cluster{"starting address":u16, "values":u16[]} {"starting address"=4272, "values"=[]}, "starting address"=w867, "values"=w873) -> (w875:cluster{"starting address":u16, "values":u16[]})
              }
              frame "多项式" {
                # "b,k,c"
                n527 = local read "多项式系数1"() -> (w888:dbl[])
                n528 = local read "量程选择"() -> (w878:enum16{"低量程", "高量程"})
                n529 = Index Array(array=w888) -> (element #1=w883:dbl, element #2=w884:dbl, element #3=w879:dbl)  [unwired: 3 in]
                n530 = Build Array(w884, w883, w879) -> (w887:dbl[])
                n531 = case shown="\"低量程\", 默认" w878 {
                  tunnel: [u16 4626 ("starting address") u16 4632 ("starting address")] -> w885
                  frame "低量程", Default {
                  }
                  frame "高量程" {
                  }
                }
                n532 = call "浮点转CDAB整形cod.vi"("浮点数"=w887) -> ("CDAB整形输出"=w886:u16[])  [unwired: 10 in]
                n533 = Bundle By Name(cluster=cluster{"starting address":u16, "values":u16[]} {"starting address"=4272, "values"=[]}, "starting address"=w885, "values"=w886) -> (w881:cluster{"starting address":u16, "values":u16[]})
              }
            }
            n534 = Enqueue Element(queue=w862, element=w865, timeout in ms (-1)=1000 ("超时毫秒(-1)")) -> ()  [unwired: 1 in, 3 out]
          }
          frame #1 {
            n535 = local write "枚举"(enum16{"读取数据", "写入数据", "读取写入DATABASE", "读取参数"}."写入数据" ("枚举")) -> ()
          }
        }
      }
      event "滴定曲线": Value Change {
        n536 = event-data() -> ()  [unwired: 1 in, 6 out]
        n537 = property on="窗格" class="Pane"("Origin"=T9 {"Horizontal"=0, "Vertical"=3200} ("原点")) -> ()  [unwired: 2 in, 2 out]
      }
      event "历史波形": Value Change {
        n538 = event-data() -> ()  [unwired: 1 in, 6 out]
        n539 = call-poly <vilib>:"Read Waveforms from File.vi"() -> ("error out"=w893:errorcluster, "first waveform in record"=w894:waveform(dbl))  [unwired: 6 in, 2 out]
        n540 = case shown="无错误" w893 {
          tunnel: w894 -> [w897 _]
          frame No Error {
            n541 = Unbundle By Name(w897) -> ("t0"=→"波形时间":timestamp, "Y"=w896:dbl[])  [unwired: 2 out]
            n542 = local write "ORP滴定曲线2"(w896) -> ()
            n543 = local write "滴定数-ORP值"(w896) -> ()
          }
          frame Error {
            n544 = One Button Dialog(message="打开失败" ("消息")) -> ()  [unwired: 1 in, 1 out]
          }
        }
      }
    }
  }
  n545 = while {
    tunnel: w34 -> [w1015]
    tunnel: w33 -> [w1014]
    tunnel: w22 -> [w1010]
    tunnel: w21 -> [w1009]
    stop <- FALSE stop-if-true
    w934 = T12 0 items=["最小二乘", "最小绝对残差", "Bisquare"] ("method")
    n546 = local read "浓度5"() -> (w903:dbl)
    n547 = local read "浓度4"() -> (w904:dbl)
    n548 = local read "浓度2"() -> (w947:dbl)
    n549 = local read "浓度3"() -> (w948:dbl)
    n550 = local read "浓度1"() -> (w946:dbl)
    n551 = local read "启用4"() -> (w900:bool)
    n552 = local read "泵滴定数3"() -> (w951:dbl)
    n553 = local read "启用3"() -> (w954:bool)
    n554 = local read "启用5"() -> (w899:bool)
    n555 = Wait (ms)(milliseconds to wait=u32 500 ("等待时间（毫秒）")) -> ()  [unwired: 1 out]
    n556 = local read "泵滴定数2"() -> (w950:dbl)
    n557 = local read "泵滴定数4"() -> (w902:dbl)
    n558 = local read "泵滴定数5"() -> (w901:dbl)
    n559 = local read "启用2"() -> (w953:bool)
    n560 = local read "泵滴定数1"() -> (w949:dbl)
    n561 = local read "启用1"() -> (w952:bool)
    n562 = Bundle By Name(cluster=T6 {"starting address"=4224, "number of holding registers"=16}, "starting address"=u16 4224, "number of holding registers"=u16 50) -> (w1069:T6)
    n563 = local read "基本量程"() -> (w917:enum16{"10mL", "20mL"})
    n564 = Build Array(w952, w953, w954, w900, w899) -> (w935:bool[])
    n565 = Multiply(x="浓度 2", y=100.0) -> (x*y=w990:dbl)
    n566 = Build Array(w946, w947, w948, w904, w903) -> (w937:dbl[])
    n567 = Build Array(w949, w950, w951, w902, w901) -> (w936:dbl[])
    n568 = Multiply(x="温度", y=10.0) -> (x*y=w993:dbl)
    n569 = local write "浓度"(w990) -> ()
    n570 = global write "COD浓度全局变量.vi" "基本量程"(w917) -> ()
    n571 = local write "温度 2"(w993) -> ()
    n572 = global write "COD浓度全局变量.vi" "跨度液浓度"("跨度液浓度") -> ()
    n573 = call "线性公式CODMn用.vi"("标液浓度"=w937, "监测浓度"=w936, "启用"=w935, "method"=w934, "模型"="模型", "精度"=4) -> ("拟合方程"=→"拟合公式":string, "r^2"=→"r^2":dbl, "slope"=→"K":dbl, "intercept"=→"b":dbl, "XY图"=→"XY图":cluster{"X Values":dbl[], "Y Values":dbl[]}[], "Polynomial Coefficients"=→"多项式系数1":dbl[])  [unwired: 8 in]
    n574 = Multiply(x="修正系数 2", y=100.0) -> (x*y=w987:dbl)
    n575 = local write "修正系数"(w987) -> ()
    n576 = disable-structure shown="禁用" {
      frame Disabled {
        n577 = global read "系统变量.vi" "自动切换量程"() -> (w1075:bool)
        n578 = local write "自动切换量程"(w1075) -> ()
      }
      frame Enabled {
      }
    }
    n579 = Enqueue Element(queue=w1015, element=w1069, error in (no error)=w1014) -> ()  [unwired: 1 in, 3 out]
    n580 = local read "Registers"() -> (w926:u16[])
    n581 = To Word Integer(number=w926) -> (16bit integer=w925:i16[])
    n582 = Index Array(array=w925, index #1=0 ("索引"), index #4=3 ("索引"), index #14=13 ("索引"), index #15=14 ("索引"), index #32=31 ("索引")) -> (element #1=w984:i16, element #2=w983:i16, element #3=w982:i16, element #4=w916:i16, element #5=→"模式（受控）":i16, element #6=→"进样管":i16, element #7=→"高锰酸钾":i16, element #8=→"草酸钠":i16, element #9=→"硫酸":i16, element #10=w924:i16, element #11=w1042:i16, element #12=w1044:i16, element #13=w915:i16, element #14=w1060:i16, element #15=w1017:i16, element #16=w940:i16, element #33=→"分":i16, element #34=→"秒":i16)  [unwired: 29 in, 16 out]
    "多列列表框" <- w940
    n583 = To Single Precision Float(number=w924) -> (single precision float=→"ORP显示":sgl)
    n584 = global write "COD测量模式全局.vi" "CODMn工作状态"(w916) -> ()
    n585 = Divide(x=w1060, y=u16 1000) -> (x/y=→"零点滴定值":dbl)
    n586 = Divide(x=w1017, y=u16 1000) -> (x/y=→"标度滴定值":dbl)
    n587 = Build Array(w984, w983, w982) -> (w985:i16[])
    n588 = global write "运行时序全局变量.vi" "多列列表框"(w940) -> ()
    n589 = Equal?(x=w915, y=u16 1) -> (x = y?=w914:bool)
    "ORP故障" <- w914
    n590 = Equal?(x=w915, y=u16 2) -> (x = y?=w913:bool)
    "温控器故障" <- w913
    n591 = Equal?(x=w915, y=u16 3) -> (x = y?=w912:bool)
    "加热故障" <- w912
    n592 = Equal?(x=w915, y=u16 4) -> (x = y?=w911:bool)
    "高锰酸钾报警" <- w911
    n593 = Equal?(x=w915, y=u16 5) -> (x = y?=w910:bool)
    "草酸钠报警" <- w910
    n594 = Equal?(x=w915, y=u16 6) -> (x = y?=w909:bool)
    "测量错误" <- w909
    n595 = Equal?(x=w915, y=u16 8) -> (x = y?=w908:bool)
    "校零错误" <- w908
    n596 = Equal?(x=w915, y=u16 7) -> (x = y?=w907:bool)
    "校标错误" <- w907
    n597 = Equal?(x=w915, y=u16 9) -> (x = y?=w906:bool)
    "进水样超量程" <- w906
    n598 = Equal?(x=w915, y=u16 10) -> (x = y?=w905:bool)
    "排液故障" <- w905
    n599 = Equal?(x=w1044, y=u16 1) -> (x = y?=→"排液标记":bool)
    n600 = Equal?(x=w916, y=u16 0) -> (x = y?=→"待机":bool)
    n601 = Equal?(x=w916, y=u16 7) -> (x = y?=→"质控样测量":bool)
    n602 = Equal?(x=w916, y=u16 1) -> (x = y?=→"水样测量":bool)
    n603 = Equal?(x=w940, y=u16 5) -> (x = y?=w1013:bool)
    n604 = Equal?(x=w916, y=u16 9) -> (x = y?=→"校标标记":bool)
    n605 = Equal?(x=w916, y=u16 6) -> (x = y?=→"平行样测量":bool)
    n606 = Equal?(x=w916, y=u16 2) -> (x = y?=→"标样核查标记":bool)
    n607 = Equal?(x=w916, y=u16 8) -> (x = y?=→"校零标记":bool)
    n608 = Divide(x=w1042, y=u16 10) -> (x/y=→"温度":dbl)
    n609 = Equal?(x=w916, y=u16 10) -> (x = y?=→"加标回收测量":bool)
    n610 = Compound Arithmetic op=OR ("复合运算")(w914, w913, w912, w911, w910, w909, w907, w908, w906, w905) -> (→"故障标记":bool)
    n611 = Bundle By Name(cluster=T3 {"ORP故障"=FALSE, "温控器故障"=FALSE, "加热故障"=FALSE, "高锰酸钾报警"=FALSE, "草酸钠报警"=FALSE, "测量错误"=FALSE, "校零错误"=FALSE, "校标错误"=FALSE, " 进水样超量程"=FALSE, "排液阀故障"=FALSE} ("报警簇"), "ORP故障"=w914, "温控器故障"=w913, "加热故障"=w912, "高锰酸钾报警"=w911, "草酸钠报警"=w910, "测量错误"=w909, "校零错误"=w908, "校标错误"=w907, "进水样超量程"=w906, "排液阀故障"=w905) -> (w1001:T3)
    "报警簇" <- w1001
    n612 = call <vilib>:"Boolean Crossing PtByPt.vi"("direction"=enum16{"either", "false-true", "true-false"}."false-true", "input"=w1013) -> ("crossing"=w1011:bool)  [unwired: 1 in]
    n613 = call "HexToDate.vi"("数组"=w985) -> ("DATE"=w980:timestamp[])  [unwired: 10 in]
    n614 = Equal?(x=w916, y=u16 3) -> (x = y?=→"零点核查标记":bool)
    n615 = feedback #1(w940) -> (w1000:i16)
    n616 = feedback-in #1(w940) -> ()
    n617 = Equal?(x=w916, y=u16 4) -> (x = y?=→"跨度核查标记":bool)
    n618 = Equal?(x=w916, y=u16 5) -> (x = y?=→"空白测试标记":bool)
    n619 = Not Equal?(x=w940, y=w1000) -> (x != y?=w999:bool)
    n620 = case shown="真" w1011 {
      tunnel: w1010 -> [_ w1173]
      tunnel: w1009 -> [_ w1168]
      frame False {
      }
      frame True {
        n621 = Bundle By Name(cluster=T6 {"starting address"=0, "number of holding registers"=0}, "starting address"=u16 4101, "number of holding registers"=u16 10) -> (w1172:T6)
        n622 = Enqueue Element(queue=w1173, element=w1172, error in (no error)=w1168) -> ()  [unwired: 1 in, 3 out]
        n623 = local write "枚举"(enum16{"读取数据", "写入数据", "读取写入DATABASE", "读取参数"}."读取写入DATABASE" ("枚举")) -> ()
      }
    }
    n624 = case shown="真" w999 {
      tunnel: w940 -> [_ w1151]
      frame False {
      }
      frame True {
        n625 = property on="多列列表框" class="MCListbox (严格)"() -> ("ItemNames"=w1145:string[][])  [unwired: 2 in, 2 out]
        n626 = Index Array(array=w1145, index (row)=w1151) -> (element=w1142:string[])  [unwired: 1 in]
        n627 = Index Array(array=w1142, index=0 ("索引")) -> (element=w1140:string)
        n628 = Array To Spreadsheet String(delimiter (Tab)="-" ("分隔符(Tab)"), array=w1142, 3:"" ("格式字符串")) -> ()  [unwired: 1 out]
        n629 = Get Date/Time In Seconds() -> (seconds since 1Jan1904=w1149:timestamp)
        n630 = Bundle(cluster="data in", "时间标识"=w1149, "参数"="CODMn" ("table输入"), "日志信息"=w1140, "流程参数"="" ("table输入")) -> (w1146:T2)
        n631 = call "流程日志字段定义.vi"("table输入"="操作日志", "data in"=w1146) -> ("table输出"=w1154:string, "columns"=w1155:string[], "data out"=w1156:T13)  [unwired: 7 in]
        n632 = call "插入数据.vi"("data"=w1156, "columns"=w1155, "database"="database3.mdb", "table"=w1154) -> ()  [unwired: 7 in, 1 out]
      }
    }
    n633 = Index Array(array=w980) -> (element=→"仪器时间":timestamp)  [unwired: 1 in]
    n634 = Get Date/Time In Seconds() -> (seconds since 1Jan1904=w979:timestamp)
    "系统时间" <- w979
    n635 = global read "COD读取DATA全局.vi" "data"() -> (w962:T5)
    n636 = Less Or Equal?(x=w940, y=u16 4) -> (x <= y?=w944:bool)
    n637 = global read "COD测量模式全局.vi" "测量模式"() -> (w961:string)
    n638 = Build Array(w979) -> (w978:timestamp[])
    n639 = Unbundle By Name(w962) -> ("时间"=w959:timestamp, "检测值"=w958:sgl, "数据标识"=w957:string)
    n640 = case shown="真" w944 {
      frame False {
      }
      frame True {
        n641 = local read "跨度核查标记"() -> (w1085:bool)
        n642 = local read "空白测试标记"() -> (w1084:bool)
        n643 = local read "加标回收测量"() -> (w1083:bool)
        n644 = local read "标样核查标记"() -> (w1090:bool)
        n645 = local read "零点核查标记"() -> (w1089:bool)
        n646 = local read "平行样测量"() -> (w1082:bool)
        n647 = local read "校零标记"() -> (w1081:bool)
        n648 = local read "校标标记"() -> (w1080:bool)
        n649 = local read "水样测量"() -> (w1091:bool)
        n650 = local read "测量模式数字"() -> (w1087:i32)
        n651 = Build Array(w1091, w1090, w1089, w1085, w1084, w1083, w1082, w1081, w1080) -> (w1088:bool[])
        n652 = case shown="4" w1087 {
          tunnel: ["水样测试" ("测量模式") "标样核查" ("测量模式") "零点核查" ("测量模式") "跨度核查" ("测量模式") "空白测试" ("测量模式") "加标回收" ("测量模式") "平行样" ("测量模式") "校零" ("测量模式") "校标" ("测量模式")] -> w1086
          frame 0, Default {
          }
          frame 1 {
          }
          frame 2 {
          }
          frame 3 {
          }
          frame 4 {
          }
          frame 5 {
          }
          frame 6 {
          }
          frame 7 {
          }
          frame 8 {
          }
        }
        n653 = for {
          tunnel: w1088 -> [w1102] mode=indexing
          i -> [w1101]
          n654 = case shown="真" w1102 {
            tunnel: w1101 -> [_ w1103]
            frame False {
            }
            frame True {
              "测量模式数字" <- w1103
            }
          }
        }
        n655 = global write "COD测量模式全局.vi" "测量模式"(w1086) -> ()
      }
    }
    n656 = Greater?(x=w940, y=u16 0) -> (0:w941:bool)
    n657 = call "DateToHex.vi"("DATE"=w978) -> ("数组"=w977:u16[])  [unwired: 10 in]
    n658 = call "DateToHex.vi"("DATE"=w980) -> ("数组"=w972:u16[])  [unwired: 10 in]
    n659 = call <vilib>:"Boolean Crossing PtByPt.vi"("direction"=enum16{"either", "false-true", "true-false"}."false-true", "input"=w941) -> ("crossing"=w939:bool)  [unwired: 1 in]
    n660 = local read "测量数据区"() -> (w963:T1)
    n661 = case shown="\"水样测试\"" w961 {
      tunnel: w963 -> [w1104 w1109 w1114 w1119 w1124 w1129 w1134 w1139]
      tunnel: [w1104 w1108 w1110 w1118 w1123 w1128 w1130 w1138] -> w960
      tunnel: w959 -> [_ w1107 w1113 w1117 w1122 w1127 w1133 w1137]
      tunnel: w958 -> [_ w1106 w1112 w1116 w1121 w1126 w1132 w1136]
      tunnel: w957 -> [_ w1105 w1111 w1115 w1120 w1125 w1131 w1135]
      frame "", Default {
      }
      frame "水样测试" {
        n662 = Bundle By Name(cluster=w1109, "水样数据时间"=w1107, "水样实测值"=w1106, "水样数据标识"=w1105) -> (w1108:T1)
      }
      frame "标样核查" {
        n663 = Bundle By Name(cluster=w1114, "跨度核查数据时间"=w1113, "跨度核查实测值"=w1112, "跨度核查数据标识"=w1111) -> (w1110:T1)
      }
      frame "零点核查" {
        n664 = Bundle By Name(cluster=w1119, "零点核查数据时间"=w1117, "零点核查实测值"=w1116, "零点核查数据标识"=w1115) -> (w1118:T1)
      }
      frame "加标回收" {
        n665 = Bundle By Name(cluster=w1124, "加标回收数据时间"=w1122, "加标回收实测值"=w1121, "加标回收数据标识"=w1120) -> (w1123:T1)
      }
      frame "平行样" {
        n666 = Bundle By Name(cluster=w1129, "平行样数据时间"=w1127, "平行样实测值"=w1126, "平行样数据标识"=w1125) -> (w1128:T1)
      }
      frame "校零" {
        n667 = Bundle By Name(cluster=w1134, "空白数据时间"=w1133, "空白实测值"=w1132, "空白数据标识"=w1131) -> (w1130:T1)
      }
      frame "校标" {
        n668 = Bundle By Name(cluster=w1139, "标样数据时间"=w1137, "标样实测值"=w1136, "标样数据标识"=w1135) -> (w1138:T1)
      }
    }
    "测量数据区" <- w960
    n669 = Index Array(array=w972, index=2 ("索引")) -> (element=w974:u16)
    n670 = case shown="真" w939 {
      frame False {
      }
      frame True {
        n671 = Get Date/Time In Seconds() -> (seconds since 1Jan1904=w1076:timestamp)
        "启动时间" <- w1076
        n672 = global read "COD测量模式全局.vi" "测量模式"() -> (w1077:string)
        n673 = case shown="\"加标回收\"" w1077 {
          tunnel: w1076 -> [w1078 w1079]
          frame "水样测试", Default {
            n674 = global write "COD测量模式全局.vi" "水样启动时间"(w1078) -> ()
          }
          frame "加标回收" {
            n675 = global write "COD测量模式全局.vi" "加标回收启动时间"(w1079) -> ()
          }
        }
      }
    }
    n676 = Index Array(array=w977, index=2 ("索引")) -> (element=w975:u16)
    n677 = Split Number(x=w974) -> (hi(x)=w968:u8)  [unwired: 1 out]
    n678 = call "CODMn报警信息.vi"("报警簇"=w1001) -> ("CODMN报警信息"=w1002:string)  [unwired: 10 in]
    n679 = Split Number(x=w975) -> (hi(x)=w971:u8)  [unwired: 1 out]
    n680 = To Byte Integer(number=w968) -> (8bit integer=w967:i8)
    n681 = To Byte Integer(number=w971) -> (8bit integer=w970:i8)
    n682 = Subtract(x=w967, y=w970) -> (x-y=w969:i8)
    n683 = feedback #2(w1002) -> (w1003:string)
    n684 = feedback-in #2(w1002) -> ()
    n685 = Not Equal?(x=w1002, y="") -> (x != y?=w1007:bool)
    n686 = Absolute Value(x=w969) -> (abs(x)=w966:i8)
    n687 = Greater Or Equal?(x=w966, y=i8 5) -> (x >= y?=w964:bool)
    n688 = Not Equal?(x=w1002, y=w1003) -> (x != y?=w1004:bool)
    n689 = disable-structure shown="禁用" {
      disable-tunnel: w964 -> [w1070 _]
      frame Disabled {
        # "自动校时"
        n690 = case shown="真" w1070 {
          tunnel: w1070 -> [_ w1071]
          frame False {
          }
          frame True {
            n691 = flat-sequence {
              tunnel: w1071 -> [_]
              frame #0 {
                n692 = property on="时间校准" class="Bool (严格)"("Val(Sgnl)"=TRUE ("时间校准")) -> ()  [unwired: 2 in, 2 out]
              }
              frame #1 {
                n693 = Wait (ms)(milliseconds to wait=u32 300 ("等待时间（毫秒）")) -> ()  [unwired: 1 out]
              }
              frame #2 {
                n694 = property on="时间校准" class="Bool (严格)"("Val(Sgnl)"=FALSE ("时间校准")) -> ()  [unwired: 2 in, 2 out]
              }
            }
          }
        }
      }
      frame Enabled {
      }
    }
    n695 = And(x=w1004, y=w1007) -> (x .and. y?=w1005:bool)
    n696 = case shown="真" w1005 {
      tunnel: w1002 -> [_ w1157]
      frame False {
      }
      frame True {
        n697 = Get Date/Time In Seconds() -> (seconds since 1Jan1904=w1159:timestamp)
        n698 = Bundle By Name(cluster=T11 {"时间标识"=timestamp(0 s since 1904-01-01), "设备"="", "日志信息"=""} ("data in"), "时间标识"=w1159, "设备"="CODMn", "日志信息"=w1157) -> (w1160:T11)
        n699 = call "报警信息字段定义.vi"("table输入"="报警信息", "data in"=w1160) -> ("table输出"=w1164:string, "columns"=w1165:string[], "data out"=w1166:T11)  [unwired: 7 in]
        n700 = call "插入数据.vi"("data"=w1166, "columns"=w1165, "database"="database3.mdb", "table"=w1164) -> ()  [unwired: 7 in, 1 out]
      }
    }
  }
  n701 = while {
    tunnel: w15 -> [w1175]
    stop <- FALSE stop-if-true
    n702 = event shown="[0] \"保存\": 鼠标按下" {
      selector: _ -> [_]
      dyn-events: _ -> [_]
      timeout: _ -> [_]
      tunnel: w1175 -> [w1195]
      event "保存": Mouse Down {
        (unwired) 1000 ("超时毫秒(-1)")
        (unwired) cluster{"starting address":u16, "values":u16[]} {"starting address"=4625, "values"=[]}
        n703 = event-data() -> ()  [unwired: 1 in, 8 out]
        n704 = call <vilib>:"Application Directory.vi"() -> ("Application Directory"=w1182:path)
        n705 = Build Path(base path=w1182, name or relative path="data\\Set.ini" ("名称或相对路径")) -> (appended path=w1180:path)
        n706 = local write "枚举"(enum16{"读取数据", "写入数据", "读取写入DATABASE", "读取参数"}."写入数据" ("枚举")) -> ()
        n707 = local read "跨度液浓度"() -> (w1185:dbl)
        n708 = call <vilib>:"Open Config Data.vi"("configuration file path"=w1180) -> ("error out"=w1178:errorcluster, "refnum"=w1179:T10)  [unwired: 8 in, 1 out]
        n709 = call-poly <vilib>:"Write Key.vi"("section"="CODMn参数" ("key"), "error in (no error)"=w1178, "value"=w1185, "key"="跨度液浓度", "refnum"=w1179) -> ("error out"=w1176:errorcluster, "refnum out"=w1177:T10)  [unwired: 4 in, 1 out]
        n710 = call <vilib>:"Close Config Data.vi"("error in (no error)"=w1176, "refnum"=w1177) -> ()  [unwired: 8 in, 2 out]
        n711 = local write "水样"("水样") -> ()
        n712 = local write "标液"("标液") -> ()
        n713 = local write "硫酸"("硫酸") -> ()
        n714 = local write "恒温时间"("恒温时间") -> ()
        n715 = local write "修正系数"("修正系数") -> ()
        n716 = local write "加标回收"("加标回收") -> ()
        n717 = local write "高锰酸钾"("高锰酸钾") -> ()
        n718 = local write "基本量程"("基本量程") -> ()
        n719 = local write "标样浓度 2"("标样浓度 2") -> ()
        n720 = local write "零点泵计量数 2"("零点泵计量数 2") -> ()
        n721 = local write "标度泵计量数 2"("标度泵计量数 2") -> ()
        n722 = local write "蒸馏水"("蒸馏水") -> ()
        n723 = local write "温度 2"("温度 2") -> ()
        n724 = local write "草酸钠"("草酸钠") -> ()
        n725 = local write "质控样"("质控样") -> ()
        n726 = Build Array("温度 2", "恒温时间", "浓度", "修正系数", "基本量程", "水样", "蒸馏水", "标液", "质控样", "加标回收", "高锰酸钾", "草酸钠", "硫酸", "零点泵计量数 2", "标度泵计量数 2", "标样浓度 2") -> (w1193:dbl[])
        n727 = Bundle By Name(cluster=cluster{"starting address":u16, "values":u16[]} {"starting address"=4272, "values"=[]}, "starting address"=u16 4272, "values"=w1193) -> (w1191:cluster{"starting address":u16, "values":u16[]})
        n728 = Enqueue Element(queue=w1195, element=w1191, timeout in ms (-1)=1000 ("超时毫秒(-1)")) -> ()  [unwired: 1 in, 3 out]
      }
    }
  }
  n729 = while {
    tunnel: w19 -> [w1225]
    tunnel: w18 -> [w1224]
    tunnel: w15 -> [w1223]
    tunnel: w34 -> [w1222]
    tunnel: w33 -> [w1221]
    tunnel: [w1211] -> w32
    tunnel: [w1220] -> w31
    tunnel: w27 -> [w1218]
    tunnel: w26 -> [w1217]
    tunnel: w22 -> [w1216]
    tunnel: w21 -> [w1215]
    tunnel: w20 -> [w1214]
    tunnel: w15 -> [w1209]
    stop <- FALSE stop-if-true
    n730 = case shown="\"读取写入DATABASE\"" "枚举" {
      tunnel: w1225 -> [w1261 w1271 w1368 w1449]
      tunnel: w1224 -> [w1260 w1267 w1367 w1448]
      tunnel: w1223 -> [_ w1270 _ _]
      tunnel: [w1227 w1269 w1370 w1443] -> w1220
      tunnel: [w1226 w1268 w1369 w1441] -> w1211
      tunnel: w1222 -> [w1258 _ _ _]
      tunnel: w1221 -> [w1254 _ _ _]
      tunnel: w1218 -> [_ _ _ w1447]
      tunnel: w1217 -> [_ _ _ w1446]
      tunnel: w1216 -> [_ _ w1366 _]
      tunnel: w1215 -> [_ _ w1365 _]
      tunnel: w1214 -> [_ w1266 _ _]
      tunnel: w1209 -> [_ _ w1317 _]
      frame "读取数据", Default {
        n731 = Dequeue Element(queue=w1258, timeout in ms (-1)=1000 ("超时毫秒(-1)"), error in (no error)=w1254) -> (element=w1257:T6)  [unwired: 3 out]
        n732 = Unbundle By Name(w1257) -> ("starting address"=w1256:u16, "number of holding registers"=w1255:u16)
        n733 = call <vilib>:"Read Holding Registers.vi"("error in (no error)"=w1260, "quantity"=w1255, "starting address"=w1256, "MB session in"=w1261) -> ("error out"=w1249:errorcluster, "Registers"=→"Registers":u16[], "MB session out"=w1252:refnum<class "MB_Master_Serial.lvclass">)  [unwired: 5 in]
        n734 = call <vilib>:"Read Coils.vi"("error in (no error)"=w1249, "quantity"=u16 8, "starting address"=u16 140, "MB session in"=w1252) -> ("error out"=w1239:errorcluster, "Coils"=w1248:bool[], "MB session out"=w1240:refnum<class "MB_Master_Serial.lvclass">)  [unwired: 5 in]
        n735 = Index Array(array=w1248) -> (element #1=→"进水样":bool, element #2=→"进蒸馏水":bool, element #3=→"进标液":bool, element #4=→"进质控样":bool, element #5=→"进加标回收样":bool, element #6=→"进高锰酸钾":bool, element #7=→"进草酸钠":bool, element #8=→"进硫酸":bool)  [unwired: 9 in, 1 out]
        n736 = call <vilib>:"Read Coils.vi"("error in (no error)"=w1239, "quantity"=u16 1, "starting address"=u16 137, "MB session in"=w1240) -> ("error out"=w1235:errorcluster, "Coils"=w1229:bool[], "MB session out"=w1236:refnum<class "MB_Master_Serial.lvclass">)  [unwired: 5 in]
        n737 = Index Array(array=w1229) -> (element=→"搅拌":bool)  [unwired: 1 in]
        n738 = call <vilib>:"Read Coils.vi"("error in (no error)"=w1235, "quantity"=u16 1, "starting address"=u16 400, "MB session in"=w1236) -> ("error out"=w1226:errorcluster, "Coils"=w1232:bool[], "MB session out"=w1227:refnum<class "MB_Master_Serial.lvclass">)  [unwired: 5 in]
        n739 = Index Array(array=w1232) -> (element=→"加热":bool)  [unwired: 1 in]
      }
      frame "写入数据" {
        n740 = flat-sequence {
          tunnel: w1271 -> [w1282]
          tunnel: w1270 -> [w1281]
          tunnel: w1267 -> [w1275]
          tunnel: w1266 -> [w1274]
          tunnel: [w1277] -> w1265
          tunnel: [w1276] -> w1264
          tunnel: [w1273] -> w1263
          tunnel: [w1272] -> w1262
          tunnel: [w1283] -> w1268
          tunnel: [w1289] -> w1269
          tunnel: w1265 -> [w1289]
          tunnel: w1264 -> [w1283]
          tunnel: w1263 -> [w1288]
          tunnel: w1262 -> [w1287]
          frame #0 {
            n741 = Dequeue Element(queue=w1281, error in (no error)=w1274) -> (queue out=w1273:refnum<queue>, element=w1280:cluster{"starting address":u16, "values":u16[]}, error out=w1272:errorcluster)  [unwired: 1 in, 1 out]
            n742 = Unbundle By Name(w1280) -> ("starting address"=w1279:u16, "values"=w1278:u16[])
            n743 = call <vilib>:"Write Multiple Registers.vi"("error in (no error)"=w1275, "values"=w1278, "starting address"=w1279, "MB session in"=w1282) -> ("error out"=w1276:errorcluster, "MB session out"=w1277:refnum<class "MB_Master_Serial.lvclass">)  [unwired: 6 in]
          }
          frame #1 {
            n744 = Get Queue Status(queue=w1288, error in (no error)=w1287) -> (# elements in queue=w1286:i32)  [unwired: 1 in, 7 out]
            n745 = Equal To 0?(x=w1286) -> (x = 0?=w1285:bool)
            n746 = case shown="真" w1285 {
              tunnel: [enum16{"读取数据", "写入数据", "读取写入DATABASE", "读取参数"}."写入数据" ("枚举") enum16{"读取数据", "写入数据", "读取写入DATABASE", "读取参数"}."读取数据" ("枚举")] -> w1284
              tunnel: w1283 -> [_ w1291]
              frame False {
              }
              frame True {
                n747 = case shown="无错误" w1291 {
                  tunnel: ["保存成功" ("消息") "保存失败" ("消息")] -> _
                  frame No Error {
                  }
                  frame Error {
                  }
                }
              }
            }
            n748 = local write "枚举"(w1284) -> ()
          }
        }
      }
      frame "读取写入DATABASE" {
        w1336 = "CODMn" ("table")
        # "高量程0-5之间会乘1.2的系数\n低量程0-2之间会乘1.1的系数"
        n749 = Dequeue Element(queue=w1366, timeout in ms (-1)=1000 ("超时毫秒(-1)"), error in (no error)=w1365) -> (element=w1373:T6)  [unwired: 3 out]
        n750 = Unbundle By Name(w1373) -> ("starting address"=w1372:u16, "number of holding registers"=w1371:u16)
        n751 = call <vilib>:"Read Holding Registers.vi"("error in (no error)"=w1367, "quantity"=w1371, "starting address"=w1372, "MB session in"=w1368) -> ("error out"=w1369:errorcluster, "Registers"=w1299:u16[], "MB session out"=w1370:refnum<class "MB_Master_Serial.lvclass">)  [unwired: 5 in]
        n752 = To Word Integer(number=w1299) -> (16bit integer=w1298:i16[])
        "DATABASE" <- w1298
        n753 = Split 1D Array(array=w1298, index=3 ("索引")) -> (first subarray=w1363:i16[], second subarray=w1353:i16[])
        n754 = global read "系统变量.vi" "运行模式"() -> (w1320:enum16{"维护模式", "常规模式", "应急模式", "质控模式"})
        n755 = case shown="\"维护模式\", 默认" w1320 {
          tunnel: ["M" ("单位") "N" ("单位") "N" ("单位") "N" ("单位")] -> w1319
          frame "维护模式", Default {
          }
          frame "常规模式" {
          }
          frame "应急模式" {
          }
          frame "质控模式" {
          }
        }
        n756 = Index Array(array=w1363) -> (element #1=w1361:i16, element #2=w1360:i16, element #3=w1359:i16)  [unwired: 3 in]
        n757 = Index Array(array=w1353) -> (element #1=w1307:i16, element #2=w1357:i16, element #3=w1356:i16, element #4=w1355:i16, element #5=w1354:i16)  [unwired: 5 in]
        n758 = Index Array(array=w1353, index=6 ("索引")) -> (element=w1351:i16)
        n759 = To Single Precision Float(number=w1307) -> (single precision float=w1309:sgl)
        n760 = Divide(x=w1309, y=sgl 100.0) -> (x/y=w1308:sgl)
        n761 = Less Or Equal?(x=w1308, y=sgl 0.01) -> (x <= y?=w1312:bool)
        n762 = case shown="真" w1312 {
          tunnel: [w1432 w1433] -> w1310
          tunnel: w1308 -> [w1432 _]
          frame False {
          }
          frame True {
            n763 = Random Number (0-1)() -> (number: 0 to 1=w1436:dbl)
            n764 = Increment(x=w1436) -> (x+1=w1434:dbl)
            n765 = Divide(x=w1434, y=sgl 100.0) -> (x/y=w1433:dbl)
          }
        }
        n766 = Build Array(w1361, w1360, w1359) -> (w1358:i16[])
        n767 = To Single Precision Float(number=w1357) -> (single precision float=w1324:sgl)
        n768 = To Single Precision Float(number=w1356) -> (single precision float=w1325:sgl)
        n769 = To Single Precision Float(number=w1355) -> (single precision float=w1326:sgl)
        n770 = To Single Precision Float(number=w1354) -> (single precision float=w1348:sgl)
        n771 = call "HexToDate.vi"("数组"=w1358) -> ("DATE"=w1362:timestamp[])  [unwired: 10 in]
        n772 = property on="基本量程" class="Enum (严格)"() -> ("Value"=w1311:enum16{"10mL", "20mL"})  [unwired: 2 in, 2 out]
        n773 = Index Array(array=w1362) -> ()  [unwired: 1 in, 1 out]
        n774 = global read "COD测量模式全局.vi" "测量模式"() -> (w1297:string)
        n775 = case shown="\"10mL\", 默认" w1311 {
          tunnel: w1310 -> [w1412 w1422]
          tunnel: [w1410 w1421] -> w1300
          frame "10mL", Default {
            n776 = Less Or Equal?(x=w1412, y=2.0) -> (x <= y?=w1415:bool)
            n777 = Greater?(x=w1412, y=0.0) -> (0:w1414:bool)
            n778 = And(x=w1415, y=w1414) -> (x .and. y?=w1411:bool)
            n779 = case shown="真" w1411 {
              tunnel: w1412 -> [w1417 w1420]
              tunnel: [w1417 w1418] -> w1410
              frame False {
              }
              frame True {
                n780 = Multiply(x=w1420, y=1.1) -> (x*y=w1418:dbl)
              }
            }
          }
          frame "20mL" {
            n781 = Greater?(x=w1422, y=0.0) -> (0:w1425:bool)
            n782 = Less Or Equal?(x=w1422, y=5.0) -> (x <= y?=w1426:bool)
            n783 = And(x=w1426, y=w1425) -> (x .and. y?=w1423:bool)
            n784 = case shown="真" w1423 {
              tunnel: w1422 -> [w1428 w1431]
              tunnel: [w1428 w1429] -> w1421
              frame False {
              }
              frame True {
                n785 = Multiply(x=w1431, y=1.2) -> (x*y=w1429:dbl)
              }
            }
          }
        }
        "COD浓度（mg/L)" <- w1300
        n786 = case shown="\"\", 默认" w1297 {
          tunnel: [0.0 w1375 w1378] -> w1296
          frame "", Default {
          }
          frame "标样核查", "校标" {
            n787 = local read "标样浓度 2"() -> (w1376:dbl)
            n788 = Divide(x=w1376, y=100.0) -> (x/y=w1375:dbl)
          }
          frame "跨度核查" {
            n789 = local read "跨度液浓度"() -> (w1378:dbl)
          }
        }
        n790 = To Single Precision Float(number=w1351) -> (single precision float=w1314:sgl)
        n791 = global read "COD测量模式全局.vi" "测量模式"() -> (w1315:string)
        n792 = global read "COD测量模式全局.vi" "测量模式"() -> (w1306:string)
        n793 = local read "启动时间"() -> (w1295:timestamp)
        n794 = Divide(x=w1348, y=sgl 1000.0) -> (x/y=w1327:sgl)
        n795 = Format Into String(format string="w%05d" ("格式字符串"), u32 1019 ("因子编码")) -> (resulting string=w1323:string)  [unwired: 2 in, 1 out]
        n796 = Not Equal?(x=w1306, y="校标") -> (x != y?=w1304:bool)
        n797 = case shown="真" w1304 {
          tunnel: w1317 -> [_ w1391]
          tunnel: w1300 -> [_ w1389]
          frame False {
            n798 = local write "枚举"(enum16{"读取数据", "写入数据", "读取写入DATABASE", "读取参数"}."读取数据" ("枚举")) -> ()
          }
          frame True {
            n799 = Greater Or Equal?(x=w1389, y=10.0) -> (x >= y?=w1387:bool)
            n800 = case shown="真" "自动切换量程" {
              tunnel: w1391 -> [_ w1394]
              tunnel: w1387 -> [_ w1393]
              frame False {
                n801 = local write "枚举"(enum16{"读取数据", "写入数据", "读取写入DATABASE", "读取参数"}."读取数据" ("枚举")) -> ()
              }
              frame True {
                n802 = case shown="真" w1393 {
                  tunnel: w1394 -> [w1396 w1404]
                  frame False {
                    # "自动切换量程"
                    n803 = local write "枚举"(enum16{"读取数据", "写入数据", "读取写入DATABASE", "读取参数"}."写入数据" ("枚举")) -> ()
                    n804 = Bundle By Name(cluster=cluster{"starting address":u16, "values":u16[]} {"starting address"=0, "values"=[]}, "starting address"=u16 4276, "values"=u16[] [0]) -> (w1399:cluster{"starting address":u16, "values":u16[]})
                    n805 = Enqueue Element(queue=w1396, element=w1399) -> ()  [unwired: 2 in, 3 out]
                  }
                  frame True {
                    n806 = local write "枚举"(enum16{"读取数据", "写入数据", "读取写入DATABASE", "读取参数"}."写入数据" ("枚举")) -> ()
                    n807 = Bundle By Name(cluster=cluster{"starting address":u16, "values":u16[]} {"starting address"=0, "values"=[]}, "starting address"=u16 4276, "values"=u16[] [1]) -> (w1405:cluster{"starting address":u16, "values":u16[]})
                    n808 = Enqueue Element(queue=w1404, element=w1405) -> ()  [unwired: 2 in, 3 out]
                  }
                }
              }
            }
          }
        }
        n809 = local read "温度"() -> (w1318:dbl)
        n810 = global read "COD测量模式全局.vi" "测量模式"() -> (w1303:string)
        n811 = Bundle(cluster=T5 {"时间"=timestamp(0 s since 1904-01-01), "测量模式"="", "数据类型"="", "检测值"=0.0, "单位"="", "数据标识"="", "因子编码"="", "标样参考值"=0.0, "ORP-A"=0.0, "ORP-B"=0.0, "ORP-K"=0.0, "COD滴定值"=0.0, "高锰酸钾滴定数"=0.0, "温度"=0.0} ("data"), "时间"=w1295, "测量模式"=w1315, "数据类型"=w1319, "检测值"=w1300, "单位"="mg/L", "数据标识"="N", "因子编码"=w1323, "标样参考值"=w1296, "ORP-A"=w1324, "ORP-B"=w1325, "ORP-K"=w1326, "COD滴定值"=w1327, "高锰酸钾滴定数"=w1314, "温度"=w1318) -> (w1316:T5)
        "data" <- w1316
        n812 = Build Array("时间", "测量模式", "数据类型", "检测值", "单位", "数据标识", "因子编码", "标样参考值", "ORPA", "ORPB", "ORPK", "COD滴定值", "高锰酸钾滴定数", "温度") -> (w1335:string[])
        "columns" <- w1335
        n813 = Equal?(x=w1303, y="校标") -> (x = y?=w1301:bool)
        n814 = global write "COD浓度全局变量.vi" "COD浓度（mg/L)"(w1300) -> ()
        n815 = global write "COD读取DATA全局.vi" "data"(w1316) -> ()
        n816 = flat-sequence {
          tunnel: w1336 -> [w1409]
          tunnel: w1335 -> [w1408]
          tunnel: w1316 -> [w1407]
          frame #0 {
            n817 = call "数据写入database.vi"("data"=w1407, "columns"=w1408, "table"=w1409) -> ()  [unwired: 8 in, 1 out]
          }
        }
        n818 = case shown="真" w1301 {
          tunnel: w1314 -> [_ w1379]
          frame False {
          }
          frame True {
            n819 = local read "当前校准"() -> (w1380:i32)
            n820 = case shown="5" w1380 {
              tunnel: w1379 -> [w1381 w1382 w1383 w1384 w1385]
              frame 1, Default {
                n821 = local write "泵滴定数1"(w1381) -> ()
              }
              frame 2 {
                n822 = local write "泵滴定数2"(w1382) -> ()
              }
              frame 3 {
                n823 = local write "泵滴定数3"(w1383) -> ()
              }
              frame 4 {
                n824 = local write "泵滴定数4"(w1384) -> ()
              }
              frame 5 {
                n825 = local write "泵滴定数5"(w1385) -> ()
              }
            }
          }
        }
        "table 输入" <- w1336
      }
      frame "读取参数" {
        n826 = Dequeue Element(queue=w1447, timeout in ms (-1)=1000 ("超时毫秒(-1)"), error in (no error)=w1446) -> (element=w1453:T6)  [unwired: 3 out]
        n827 = local write "枚举"(enum16{"读取数据", "写入数据", "读取写入DATABASE", "读取参数"}."读取数据" ("枚举")) -> ()
        n828 = Unbundle By Name(w1453) -> ("starting address"=w1452:u16, "number of holding registers"=w1451:u16)
        n829 = local read "读取KB值"() -> (w1442:bool)
        n830 = call <vilib>:"Read Holding Registers.vi"("error in (no error)"=w1448, "quantity"=w1451, "starting address"=w1452, "MB session in"=w1449) -> ("error out"=w1441:errorcluster, "Registers"=w1445:u16[], "MB session out"=w1443:refnum<class "MB_Master_Serial.lvclass">)  [unwired: 5 in]
        "读取参数" <- w1445
        n831 = case shown="真" w1442 {
          tunnel: w1445 -> [w1463 w1488]
          tunnel: w1441 -> [_ w1490]
          frame False {
            n832 = Index Array(array=w1463) -> (element #1=w1457:u16, element #2=w1476:u16, element #3=w1475:u16, element #4=w1455:u16, element #5=w1474:u16, element #6=w1473:u16, element #7=w1472:u16, element #8=w1471:u16, element #9=w1470:u16, element #10=w1469:u16, element #11=w1468:u16, element #12=w1467:u16, element #13=w1466:u16, element #14=w1465:u16, element #15=w1464:u16, element #16=w1462:u16)  [unwired: 16 in]
            n833 = local write "浓度"(w1475) -> ()
            n834 = local write "水样"(w1473) -> ()
            n835 = local write "硫酸"(w1466) -> ()
            n836 = local write "标液"(w1471) -> ()
            n837 = Divide(x=w1457, y=u16 10) -> (x/y=w1458:dbl)
            n838 = local write "草酸钠"(w1467) -> ()
            n839 = local write "蒸馏水"(w1472) -> ()
            n840 = local write "质控样"(w1470) -> ()
            n841 = local write "恒温时间"(w1476) -> ()
            n842 = local write "基本量程"(w1474) -> ()
            n843 = local write "加标回收"(w1469) -> ()
            n844 = local write "高锰酸钾"(w1468) -> ()
            n845 = local write "零点泵计量数 2"(w1465) -> ()
            n846 = local write "标度泵计量数 2"(w1464) -> ()
            n847 = Divide(x=w1455, y=u16 100) -> (x/y=w1454:dbl)
            n848 = Divide(x=w1462, y=u16 100) -> (x/y=w1461:dbl)
            n849 = local write "温度"(w1458) -> ()
            n850 = local write "修正系数 2"(w1454) -> ()
            n851 = local write "浓度 2"(w1461) -> ()
          }
          frame True {
            (unwired) 9 ("索引")
            n852 = case shown="错误" w1490 {
              tunnel: ["读取成功" ("消息") "读取失败" ("消息")] -> w1489
              frame No Error {
              }
              frame Error {
              }
            }
            n853 = Array Subset(array=w1488, index=10 ("索引"), length=12 ("长度")) -> (w1485:u16[])
            n854 = call "浮点CDAB转换COD.vi"("数组"=w1485) -> ("数组 2"=w1484:sgl[])  [unwired: 10 in]
            n855 = One Button Dialog(message=w1489) -> ()  [unwired: 1 in, 1 out]
            n856 = Array To Cluster(array=w1484) -> (cluster=w1483:T14)
            n857 = local read "量程选择"() -> (w1477:enum16{"低量程", "高量程"})
            n858 = case shown="\"高量程\"" w1477 {
              tunnel: w1483 -> [w1494 w1498]
              tunnel: [w1493 w1497] -> w1480
              tunnel: [w1492 w1496] -> w1479
              tunnel: [w1491 w1495] -> w1478
              frame "低量程", Default {
                n859 = Unbundle By Name(w1494) -> ("数组 2[2]"=w1493:sgl, "数组 2[0]"=w1492:sgl, "数组 2[1]"=w1491:sgl)
              }
              frame "高量程" {
                n860 = Unbundle By Name(w1498) -> ("数组 2[5]"=w1497:sgl, "数组 2[3]"=w1496:sgl, "数组 2[4]"=w1495:sgl)
              }
            }
            n861 = Bundle By Name(cluster=cluster{"X^2":dbl, "X":dbl, "b":dbl} {"X^2"=0.0, "X"=0.0, "b"=0.0} ("方程系数"), "X^2"=w1480, "X"=w1479, "b"=w1478) -> (w1481:cluster{"X^2":dbl, "X":dbl, "b":dbl})
            n862 = local write "方程系数"(w1481) -> ()
          }
        }
      }
    }
    n863 = Unbundle By Name(w1211) -> ("status"=w1212:bool)
    n864 = Not(x=w1212) -> (.not. x?=→"通讯状态":bool)
  }
  n865 = call <vilib>:"Application Directory.vi"() -> ("Application Directory"=w11:path)
  n866 = Build Path(base path=w11, name or relative path="data\\Set.ini" ("名称或相对路径")) -> (appended path=w9:path)
  n867 = call <vilib>:"Open Config Data.vi"("configuration file path"=w9) -> ("error out"=w5:errorcluster, "refnum"=w6:T10)  [unwired: 8 in, 1 out]
  n868 = call-poly <vilib>:"Read Key.vi"("section"="CODMn参数" ("key"), "error in (no error)"=w5, "key"="跨度液浓度", "refnum"=w6) -> ("error out"=w3:errorcluster, "value"=w2:dbl, "refnum out"=w4:T10)  [unwired: 4 in, 1 out]
  n869 = local write "跨度液浓度"(w2) -> ()
  n870 = call <vilib>:"Close Config Data.vi"("error in (no error)"=w3, "refnum"=w4) -> ()  [unwired: 8 in, 2 out]
  n871 = call-dynamic "Close Session.vi"("error in (no error)"=w32, "MB_Serial session"=w31) -> ()  [unwired: 9 in, 1 out]
